vi "laneleftright3.vi"() -> (2 "Coeff right":dbl[](array[numeric]), 3 "Coeff left":dbl[](array[numeric]))   [LabVIEW 2015]
uses:
  <vilib>/Analysis/7linalg.llb/Solve Linear Equations (single right hand).vi
  <vilib>/Analysis/baseanly.llb/Solve Linear Equations By Cholesky.vi
  <vilib>/Analysis/baseanly.llb/Real Matrix to Compact Array.vi
  <vilib>/Analysis/baseanly.llb/Real Compact Tri-Matrix Linear Eqs.vi
  G_LCM.vi
  <vilib>/Analysis/polynomials.llb/1D Polynomial Evaluation (DBL).vi
  G_SEN.vi
  G_ALL.vi
  <vilib>/Analysis/7linalg.llb/Solve Linear Eqs (General).vi
  <vilib>/Analysis/7linalg.llb/Solve Linear Eqs (Gen, single right hand).vi
  <vilib>/Analysis/polynomials.llb/nth Derivative of Polynomial (DBL).vi
  <vilib>/Analysis/polynomials.llb/Polynomial Roots (DBL).vi
  <vilib>/Analysis/polynomials.llb/Scalar Polynomial Evaluation (DBL).vi
  <vilib>/Analysis/1siggen.llb/Ramp Pattern by Delta.vi
  <vilib>/Analysis/NI_AALPro.lvlib
  <vilib>/Analysis/NI_AALBase.lvlib
panel:
  in  "y 2":dbl
  out "fractional index or x 2":dbl
  out "fractional index or x":dbl
  out "range 3":dbl[][](graph)
  out "map_dist":dbl[](array[numeric])
  out "lane_track":dbl[][](array[numeric])
  out "map_track":dbl[][](array[numeric])
  out "lane dist":dbl[](array[numeric])
  out "y_shift":dbl
  out "x_shift":dbl
  out "range 2":dbl[][](graph)
  out "range":dbl[](graph)
  in  "gain":dbl=0.5 min=-1.0 max=1.0
  out "Lane_C_M":dbl[](array[numeric])=[0.8601491478953653, 0.8717844136967624, 0.882947592858927, 0.8936326403234123, 0.9038337699485205, 0.9135454576426009, 0.9227624443554423, 0.9314797389261423, 0.9396926207859084, 0.9473966425143293, 0.9545876322477319, 0.9612616959383189, 0.9674152194628639, 0.9730448705798238, 0.9781476007338057, 0.9827206467064133, 0.9867615321125792, 0.9902680687415704, 0.993238357741943, 0.9956707906498045, 0.9975640502598242, 0.9989171113385246, 0.9997292411794617, 1.0, 0.9997292411794617, 0.9989171113385246, 0.9975640502598242, 0.9956707906498045, 0.993238357741943, 0.9902680687415704, 0.9867615321125792, 0.9827206467064133]
  out "ratio(-1:left1:right)":dbl
  out "NaN/Path/Refnum?":bool
  out "Rleft":dbl
  out "Rright":dbl
  in  "poly":i32=2 min=1 max=4 step=1
  out "Coeff stop":dbl[](array[numeric])
  out "y_end":dbl[](array[numeric])=[0.8601491478953653, 0.8717844136967624, 0.882947592858927, 0.8936326403234123, 0.9038337699485205, 0.9135454576426009, 0.9227624443554423, 0.9314797389261423, 0.9396926207859084, 0.9473966425143293, 0.9545876322477319, 0.9612616959383189, 0.9674152194628639, 0.9730448705798238, 0.9781476007338057, 0.9827206467064133, 0.9867615321125792, 0.9902680687415704, 0.993238357741943, 0.9956707906498045, 0.9975640502598242, 0.9989171113385246, 0.9997292411794617, 1.0, 0.9997292411794617, 0.9989171113385246, 0.9975640502598242, 0.9956707906498045, 0.993238357741943, 0.9902680687415704, 0.9867615321125792, 0.9827206467064133]
  in  "iter":i32=5
  out "Waveform Graph":dbl[](graph)
  out "w":dbl[](array[numeric])
  out "XY Graph 4":cluster{"Y":dbl[], "Y":dbl[]}[](graph)=[{"Y"=array[3210 elements], "Y"=array[3210 elements]}, {"Y"=[-0.0, 0.001154394197769193, 0.004617650635850623, 0.010389990872226917, 0.018471784248973222, 0.02886354801042046, 0.041565947468740205, 0.056579796217107514, 0.0739060563904701, 0.0935458389742223, 0.11550040416098284, 0.13977116175580306, 0.16635967162997645, 0.19526764422393228, 0.2264969410994837, 0.26004957554195585, 0.2959277132125635, 0.3341336728515216, 0.374669927032528, 0.417539102969144, 0.4627439833735707, 0.5102875073687159, 0.560172771454063, 0.6124030305261954, 0.6669816989546717, 0.7239123517142048, 0.7831987255740245, 0.8448447203451934, 0.9088544001870815, 0.975231994973953, 1.0439819017227023, 1.1151086860829622, 1.1886170838907617, 1.2645120027869723, 1.342798523901962, 1.42348190360768, 1.5065675753387922, 1.592061151484188, 1.6799684253507792, 1.770295373200753, 1.8630481563645134, 1.9582331234307588, 2.0558568125157564, 2.1559259536137603, 2.258447471030621], "Y"=[0.0, 0.5, 1.0, 1.5, 2.0, 2.5, 3.0, 3.5, 4.0, 4.5, 5.0, 5.5, 6.0, 6.5, 7.0, 7.5, 8.0, 8.5, 9.0, 9.5, 10.0, 10.5, 11.0, 11.5, 12.0, 12.5, 13.0, 13.5, 14.0, 14.5, 15.0, 15.5, 16.0, 16.5, 17.0, 17.5, 18.0, 18.5, 19.0, 19.5, 20.0, 20.5, 21.0, 21.5, 22.0]}, {"Y"=[0.362252581831572], "Y"=[-0.8199241909738847]}, {"Y"=array[210 elements], "Y"=array[210 elements]}, {"Y"=[-0.925, -0.925, -0.925, -0.6775, -0.6775, -0.925, -0.925, -0.925, -0.925, -0.6775, -0.6775, -0.925, -0.925, -0.925, 0.9025, 0.9025, 0.9025, 0.6775, 0.6775, 0.9025, 0.9025, 0.9025, 0.9025, 0.6775, 0.6775, 0.9025, 0.9025, 0.9025, -0.925], "Y"=[-0.75, -0.224, 0.224, 0.224, -0.224, -0.224, 0.224, 2.415, 2.885, 2.885, 2.415, 2.415, 2.885, 3.5, 3.5, 2.885, 2.415, 2.415, 2.885, 2.885, 2.415, 0.224, -0.224, -0.224, 0.224, 0.224, -0.224, -0.75, -0.75]}, {"Y"=[0.171875, 0.15377271904051304, 0.1346290179491043, 0.11445423440635205, 0.09325870609283447, 0.07105277068912982, 0.04784676587581635, 0.02365102933347224, -0.0015241012573242174, -0.02766828821599482, -0.05477119386196136, -0.08282248051464558, -0.11181181049346922, -0.14172884611785413, -0.17256324970722198, -0.20430468358099463, -0.23694281005859374, -0.27046729145944115, -0.30486779010295867, -0.340133968308568, -0.3762554883956909, -0.41322201268374914, -0.4510232034921646, -0.4896487231403589], "Y"=[0.0, 0.5, 1.0, 1.5, 2.0, 2.5, 3.0, 3.5, 4.0, 4.5, 5.0, 5.5, 6.0, 6.5, 7.0, 7.5, 8.0, 8.5, 9.0, 9.5, 10.0, 10.5, 11.0, 11.5]}, {"Y"=[1.796875, 1.778772719040513, 1.7596290179491043, 1.739454234406352, 1.7182587060928345, 1.6960527706891297, 1.6728467658758164, 1.6486510293334722, 1.6234758987426758, 1.5973317117840051, 1.5702288061380387, 1.5421775194853544, 1.513188189506531, 1.483271153882146, 1.452436750292778, 1.4206953164190055, 1.3880571899414063, 1.354532708540559, 1.3201322098970414, 1.284866031691432, 1.248744511604309, 1.2117779873162509, 1.1739767965078354, 1.135351276859641, 1.0959117660522462, 1.0556686017662287, 1.014632121682167, 0.9728126634806396, 0.9302205648422242, 0.8868661634474992], "Y"=[0.0, 0.5, 1.0, 1.5, 2.0, 2.5, 3.0, 3.5, 4.0, 4.5, 5.0, 5.5, 6.0, 6.5, 7.0, 7.5, 8.0, 8.5, 9.0, 9.5, 10.0, 10.5, 11.0, 11.5, 12.0, 12.5, 13.0, 13.5, 14.0, 14.5]}, {"Y"=[-1.453125, -1.471227280959487, -1.4903709820508957, -1.510545765593648, -1.5317412939071655, -1.5539472293108703, -1.5771532341241836, -1.6013489706665278, -1.6265241012573242, -1.6526682882159949, -1.6797711938619613, -1.7078224805146456, -1.736811810493469, -1.766728846117854, -1.797563249707222, -1.8293046835809945, -1.8619428100585937, -1.895467291459441, -1.9298677901029586], "Y"=[0.0, 0.5, 1.0, 1.5, 2.0, 2.5, 3.0, 3.5, 4.0, 4.5, 5.0, 5.5, 6.0, 6.5, 7.0, 7.5, 8.0, 8.5, 9.0]}, {"Y"=[0.171875, 0.2568230007600336, 0.3384052130063493, 0.44574342526006827, 0.5205081969556753, 0.5917680690742042, 0.659409530134929, 0.7229937549325056, 0.7835496148685115, 0.8405449546633443, 0.9258576868463875], "Y"=[-20.239964538708662, -19.725637940364884, -19.211158961966362, -18.6998967366845, -18.19022720070031, -17.681887266143153, -17.17615515566314, -16.67683575591291, -16.176265245349786, -15.679082775270938, -15.183754484614711]}, {"Y"=[7.134647485270904], "Y"=[38.71960961082238]}, {"Y"=array[980 elements], "Y"=array[980 elements]}, {"Y"=[], "Y"=[]}]
  out "y":dbl[](array[numeric])
  out "x":dbl[](array[numeric])
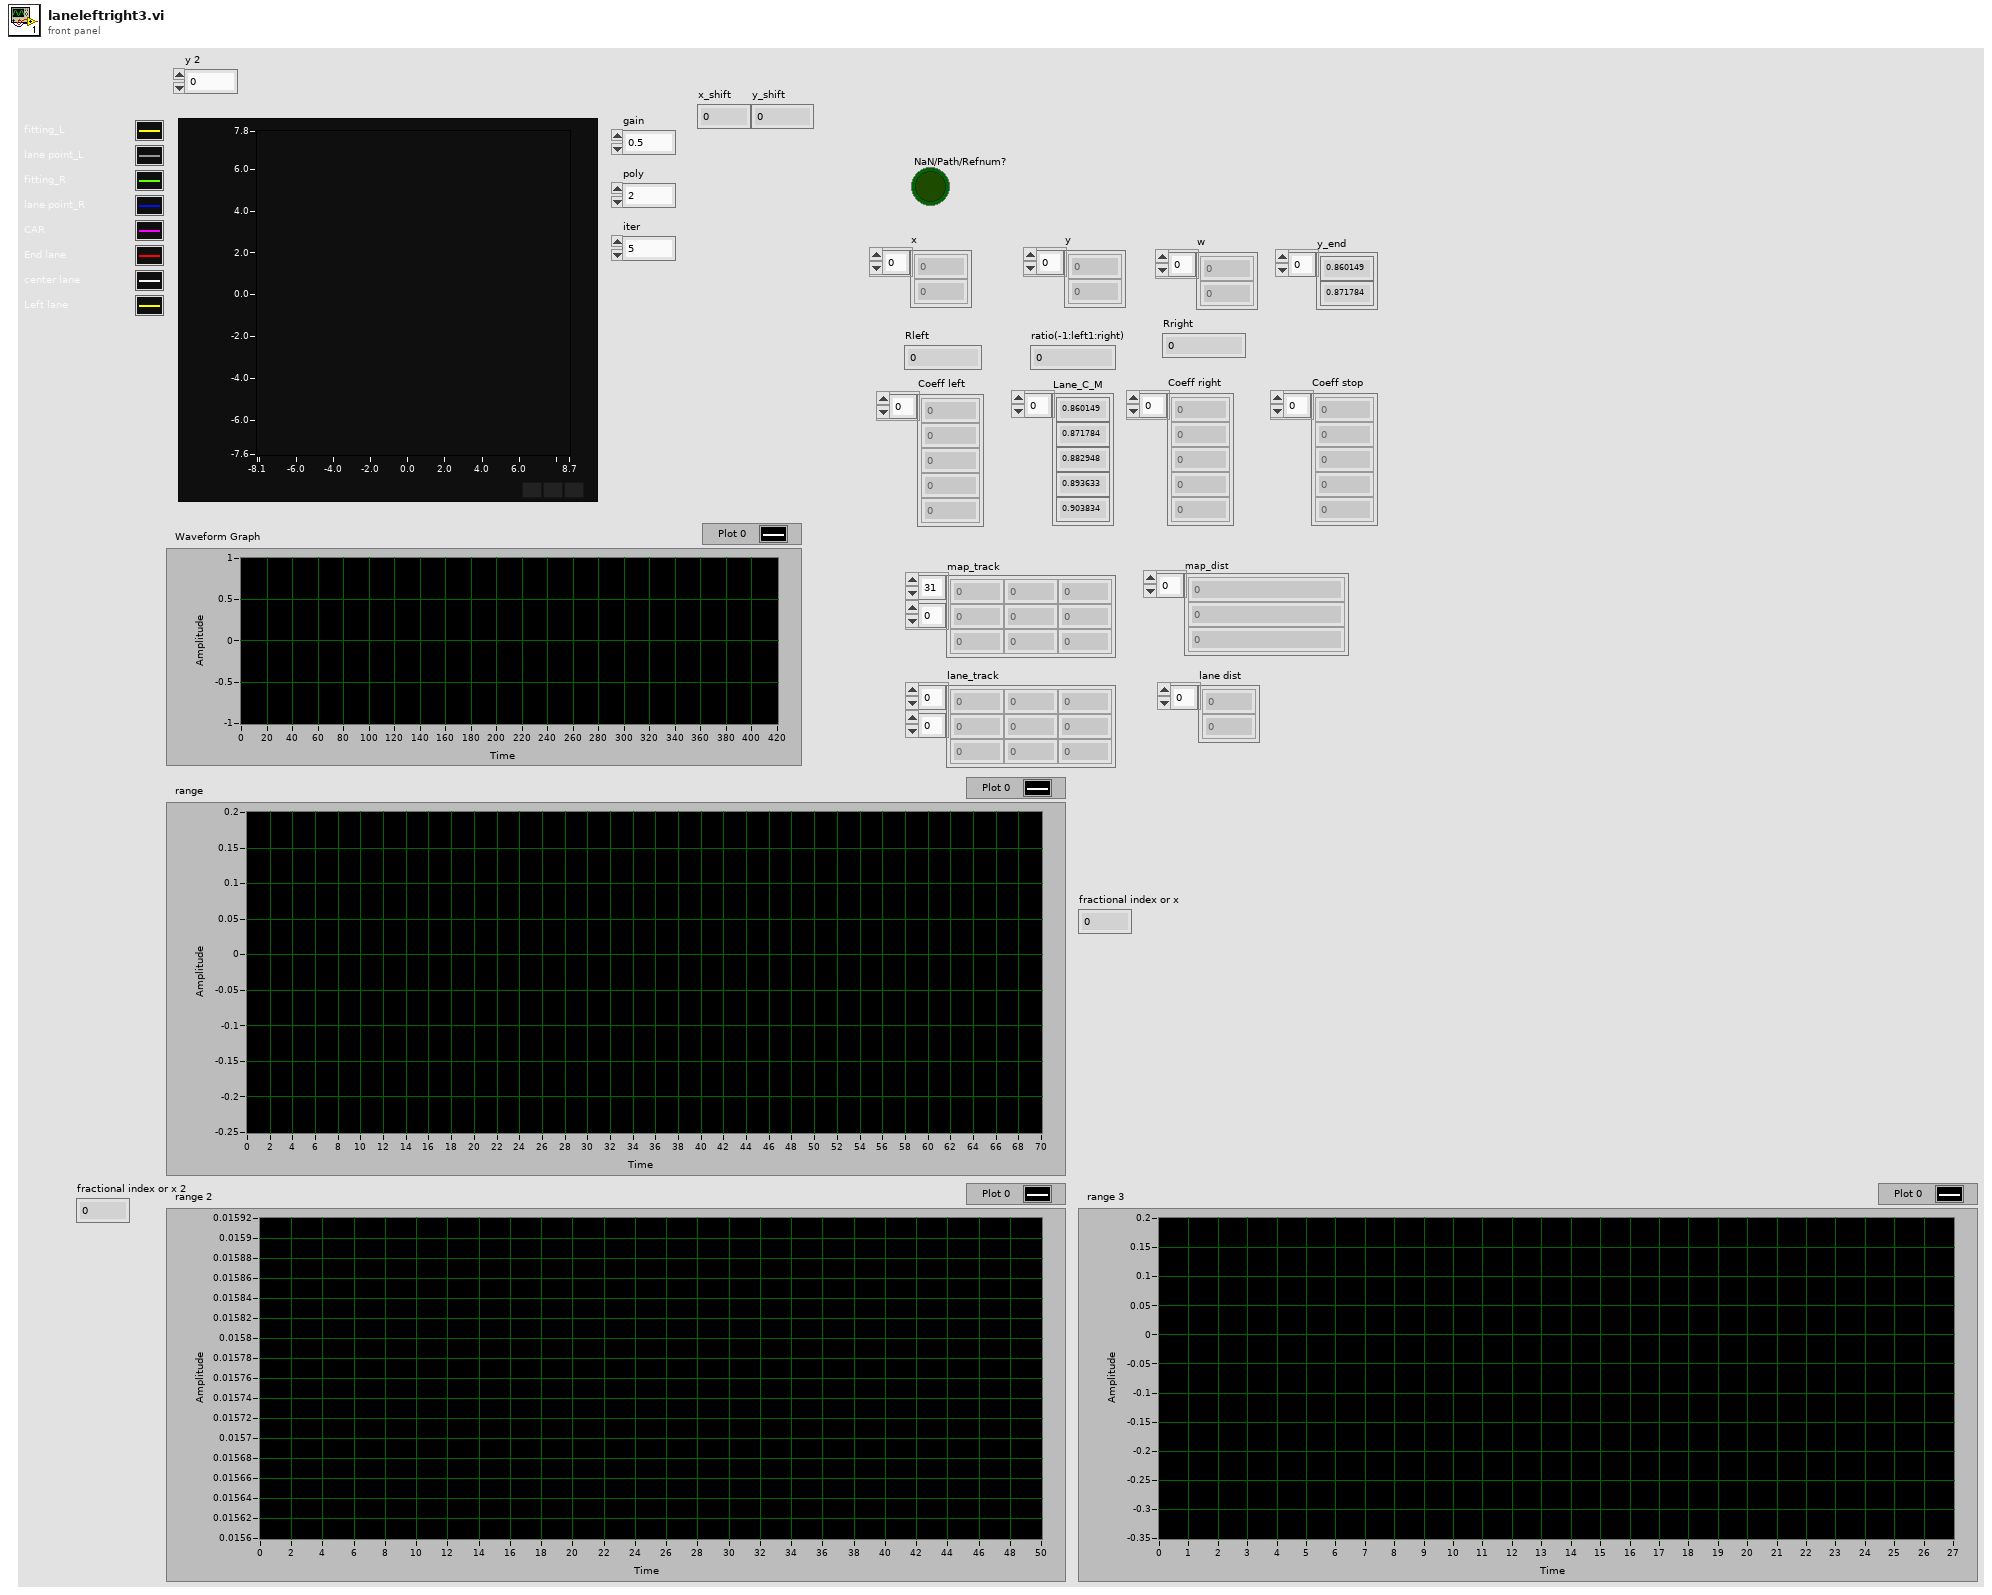
[diagram p1: front panel]
types:
  T1 = cluster{"hash":i64, "sys time":i64, "size":i64, "x":dbl[], "y":dbl[]}
  T2 = cluster{"delta":bool, "Rotational position":dbl, "Rotational position":dbl}[]
  T3 = cluster{"C_Wheel base":dbl, "ratio_steer":dbl, "Overall width":dbl, "af":dbl, "turn radius":dbl, "eval":dbl, "ap":dbl, "an":dbl, "Vmax":dbl, "mu":dbl, "Vlast":dbl}
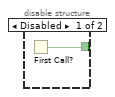
[diagram p2: hidden frame]
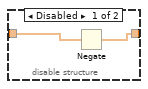
[diagram p3: hidden frame]
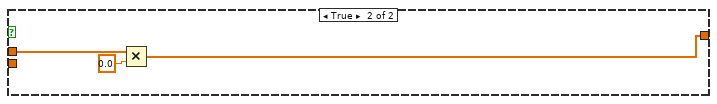
[diagram p4: hidden frame]
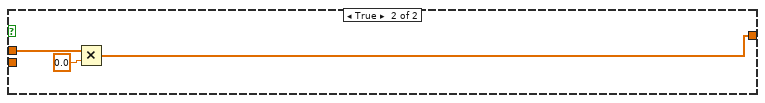
[diagram p5: hidden frame]
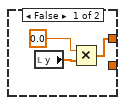
[diagram p6: hidden frame]
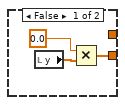
[diagram p7: hidden frame]
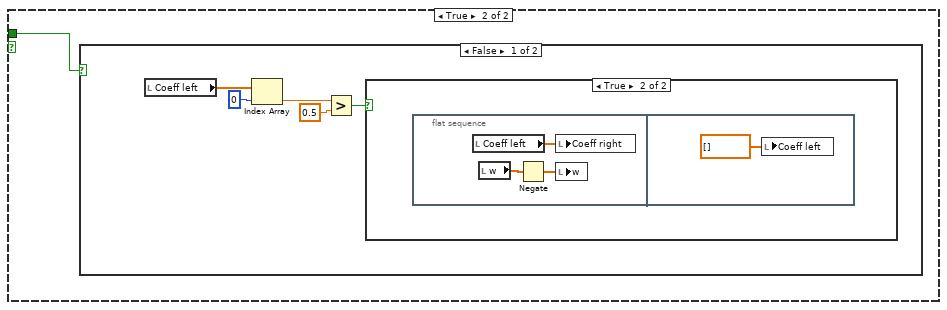
[diagram p12: hidden frame]
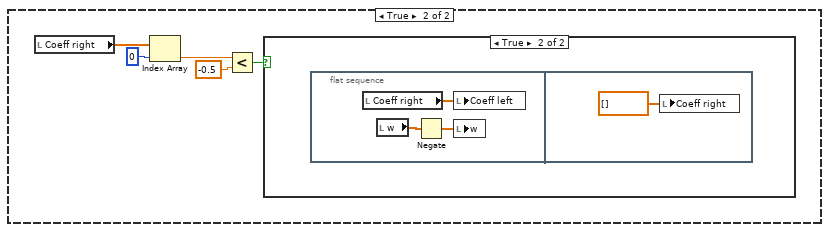
[diagram p14: hidden frame]
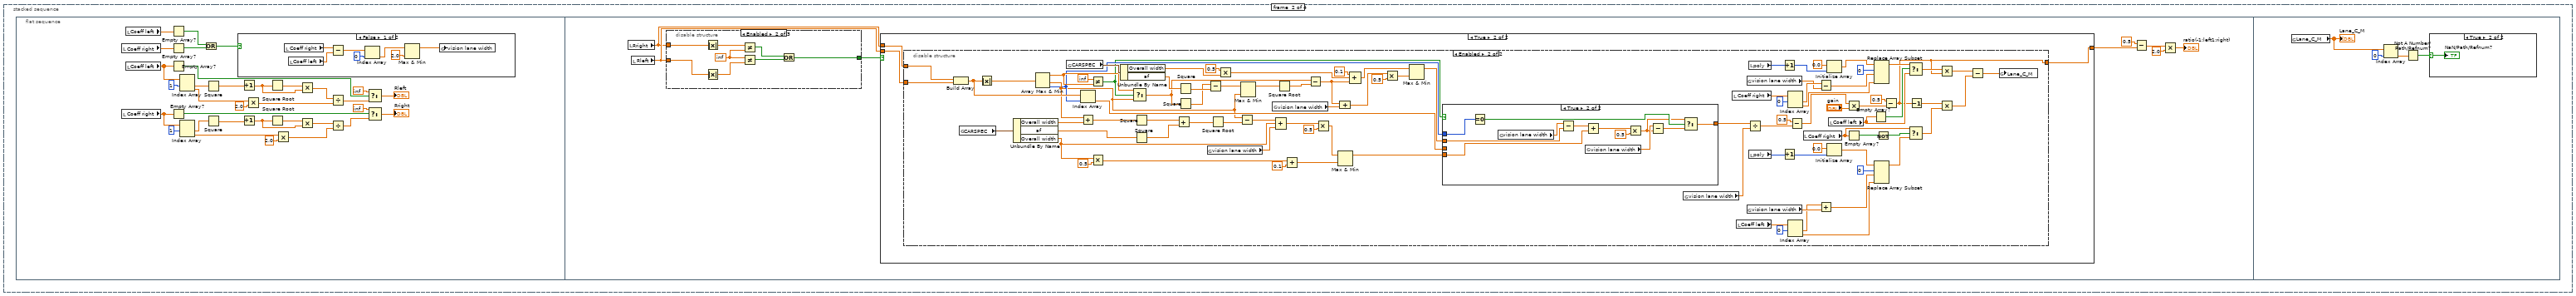
[diagram p16: hidden frame]
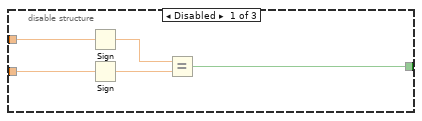
[diagram p18: hidden frame]
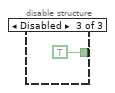
[diagram p19: hidden frame]
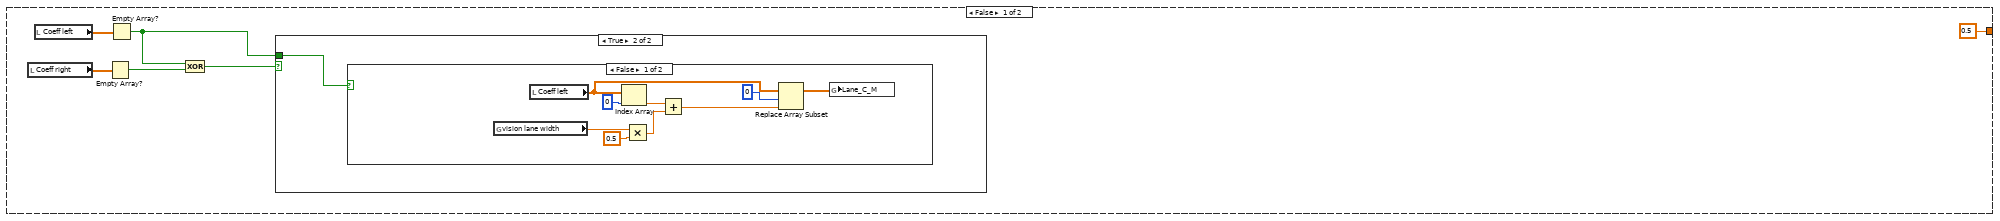
[diagram p20: hidden frame]
diagram:
  n1 = disable-structure shown="Enabled" {
    disable-tunnel: [w2 _] -> w1
    frame Disabled {
      n2 = First Call?() -> (First Call?: T/F=w2:bool)
    }
    frame Enabled {
    }
  }
  n3 = case shown="False" w1 {
    frame False {
      n4 = stacked-sequence {
        frame #0 {
          n5 = flat-sequence {
            frame #0 {
              n6 = global read "G_LCM.vi" "VISION_LANE_PT"() -> (w3:T1)
              n7 = Unbundle By Name(w3) -> ("x"=w20:dbl[], "y"=w14:dbl[])
              n8 = disable-structure shown="Enabled" {
                disable-tunnel: w20 -> [w23 w24]
                disable-tunnel: [w22 w24] -> w21
                frame Disabled {
                  n9 = Negate(x=w23) -> (-x=w22:dbl[])
                }
                frame Enabled {
                }
              }
              n10 = In Range and Coerce(upper limit=10.0 ("delta"), x=w14, lower limit=-10.0) -> (In Range?=w12:bool[])  [unwired: 1 out]
              n11 = Build Cluster Array(w12, w21, w14) -> (w10:T2)
              n12 = Sort 1D Array(array=w10) -> (sorted array=w11:T2)
              n13 = Reverse 1D Array(array=w11) -> (reversed array=w5:T2)
              n14 = for {
                tunnel: w5 -> [w28] mode=indexing
                tunnel: [w27] -> w7 mode=indexing
                tunnel: [w26] -> w8 mode=indexing
                tunnel: [w25] -> w15 mode=indexing
                n15 = Unbundle(w28) -> ("delta"=w25:bool, "Rotational position"=w27:dbl, "Rotational position"=w26:dbl)
              }
              n16 = Boolean To (0,1)(Boolean=w15) -> (0, 1=w6:i16[])
              n17 = Add Array Elements(numeric array=w6) -> (sum=w16:i16)
              n18 = Delete From Array(array=w7, length=w16, index=0) -> (deleted portion=→"x":dbl[])  [unwired: 1 out]
              n19 = Delete From Array(array=w8, length=w16, index=0) -> (deleted portion=→"y":dbl[])  [unwired: 1 out]
            }
            frame #1 {
              n20 = local read "Coeff left"() -> (w60:dbl[])
              n21 = local read "Coeff right"() -> (w59:dbl[])
              n22 = Empty Array?(array=w60) -> (empty?=w61:bool)
              n23 = Empty Array?(array=w59) -> (empty?=w62:bool)
              n24 = local read "y"() -> (w57:dbl[])
              n25 = case shown="False" w61 {
                tunnel: w57 -> [w83 w91]
                tunnel: w60 -> [w80 _]
                tunnel: [w78 w90] -> w58
                frame False {
                  n26 = call-poly <vilib>:"Polynomial Evaluation.vi"("P(x)"=w80, "A"=w83) -> ("P(A)"=w82:dbl[])  [unwired: 1 out]
                  n27 = local read "x"() -> (w81:dbl[])
                  n28 = Subtract(x=w82, y=w81) -> (x-y=w87:dbl[])
                  n29 = Absolute Value(x=w87) -> (abs(x)=w86:dbl[])
                  n30 = Negate(x=w86) -> (-x=w85:dbl[])
                  n31 = Add(x=w85, y=1.0) -> (x+y=w89:dbl[])
                  n32 = Max & Min(x=0.0, y=w89) -> (max(x,y)=w79:dbl[])  [unwired: 1 out]
                  n33 = Negate(x=w79) -> (-x=w78:dbl[])
                }
                frame True {
                  n34 = Multiply(x=w91, y=0.0) -> (x*y=w90:dbl[])
                }
              }
              n35 = local read "x"() -> (w29:dbl[])
              n36 = local read "y"() -> (w63:dbl[])
              n37 = local read "y"() -> (w30:dbl[])
              n38 = case shown="False" w62 {
                tunnel: [w72 w75] -> w55
                tunnel: w59 -> [w71 _]
                tunnel: w63 -> [w64 w76]
                frame False {
                  n39 = call-poly <vilib>:"Polynomial Evaluation.vi"("P(x)"=w71, "A"=w64) -> ("P(A)"=w69:dbl[])  [unwired: 1 out]
                  n40 = local read "x"() -> (w70:dbl[])
                  n41 = Subtract(x=w69, y=w70) -> (x-y=w65:dbl[])
                  n42 = Absolute Value(x=w65) -> (abs(x)=w66:dbl[])
                  n43 = Negate(x=w66) -> (-x=w67:dbl[])
                  n44 = Add(x=w67, y=1.0) -> (x+y=w73:dbl[])
                  n45 = Max & Min(x=0.0, y=w73) -> (max(x,y)=w72:dbl[])  [unwired: 1 out]
                }
                frame True {
                  n46 = Multiply(x=w76, y=0.0) -> (x*y=w75:dbl[])
                }
              }
              n47 = Subtract(x=w29, y=6.0) -> (x-y=w33:dbl[])
              n48 = Subtract(x=w30, y=0.0) -> (x-y=w42:dbl[])
              n49 = Subtract(x=w29, y=-6.0) -> (x-y=w35:dbl[])
              n50 = Square(x=w35) -> (x^2=w34:dbl[])
              n51 = Square(x=w33) -> (x^2=w43:dbl[])
              n52 = Square(x=w42) -> (x^2=w44:dbl[])
              n53 = Add(x=w34, y=w44) -> (x+y=w50:dbl[])
              n54 = Add(x=w44, y=w43) -> (x+y=w45:dbl[])
              n55 = In Range and Coerce(upper limit=36.0, x=w50, lower limit=4.0) -> (In Range?=w52:bool[])  [unwired: 1 out]
              n56 = In Range and Coerce(upper limit=36.0, x=w45, lower limit=4.0) -> (In Range?=w51:bool[])  [unwired: 1 out]
              n57 = Boolean To (0,1)(Boolean=w52) -> (0, 1=w53:i16[])
              n58 = Boolean To (0,1)(Boolean=w51) -> (0, 1=w54:i16[])
              n59 = Multiply(x=i16 -1, y=w53) -> (x*y=w38:i16[])
              n60 = Add(x=w38, y=w54) -> (x+y=w40:i16[])
              n61 = Multiply(x=w40, y=1.0 ("element")) -> (x*y=w56:dbl[])
              n62 = Compound Arithmetic op=ADD(w56, w55, w58) -> (→"w":dbl[])
            }
            frame #2 {
              n63 = for {
                N: "iter" -> [_]
                tunnel: "poly" -> [w96]
                n64 = flat-sequence {
                  tunnel: [w110] -> w102
                  tunnel: w96 -> [w103]
                  tunnel: [w103] -> w95
                  tunnel: [w141] -> w101
                  tunnel: w102 -> [w141]
                  tunnel: [w138] -> w99
                  tunnel: w95 -> [w131]
                  tunnel: w101 -> [w203]
                  tunnel: [w203] -> w100
                  tunnel: w99 -> [w202]
                  tunnel: [w202] -> w98
                  tunnel: [w173] -> w97
                  tunnel: w100 -> [w211]
                  tunnel: w98 -> [w210]
                  tunnel: w97 -> [w209]
                  frame #0 {
                    n65 = local read "w"() -> (w112:dbl[])
                    n66 = Greater?(x=w112, y=0.99) -> (0:w104:bool[])
                    n67 = Boolean To (0,1)(Boolean=w104) -> (0, 1=w105:i16[])
                    n68 = Add Array Elements(numeric array=w105) -> (sum=w108:i16)
                    n69 = Greater?(x=w108, y=i16 50) -> (0:w106:bool)
                    n70 = case shown="True" w106 {
                      tunnel: [w114 w121] -> w110
                      tunnel: [_ w120] -> w109
                      tunnel: w105 -> [_ w117]
                      tunnel: w103 -> [_ w116]
                      frame False {
                        n71 = local read "y"() -> (w115:dbl[])
                        n72 = Multiply(x=0.0, y=w115) -> (x*y=w114:dbl[])
                      }
                      frame True {
                        n73 = local read "x"() -> (w118:dbl[])
                        n74 = local read "y"() -> (w119:dbl[])
                        n75 = call <vilib>:"General Polynomial Fit Coefficients.vi"("Y"=w118, "polynomial order"=w116, "X"=w119, "Weight"=w117) -> ("Polynomial Coefficients"=w120:dbl[])  [unwired: 10 in, 1 out]
                        n76 = local read "y"() -> (w130:dbl[])
                        n77 = call-poly <vilib>:"Polynomial Evaluation.vi"("P(x)"=w120, "A"=w130) -> ("P(A)"=w129:dbl[])  [unwired: 1 out]
                        n78 = local read "x"() -> (w128:dbl[])
                        n79 = Subtract(x=w129, y=w128) -> (x-y=w127:dbl[])
                        n80 = Absolute Value(x=w127) -> (abs(x)=w126:dbl[])
                        n81 = Negate(x=w126) -> (-x=w125:dbl[])
                        n82 = Add(x=w125, y=1.0) -> (x+y=w122:dbl[])
                        n83 = Max & Min(x=0.0, y=w122) -> (max(x,y)=w121:dbl[])  [unwired: 1 out]
                      }
                    }
                    "Coeff right" <- w109
                  }
                  frame #1 {
                    n84 = local read "w"() -> (w139:dbl[])
                    n85 = Less?(x=w139, y=-0.99) -> (x < y?=w134:bool[])
                    n86 = Boolean To (0,1)(Boolean=w134) -> (0, 1=w132:i16[])
                    n87 = Add Array Elements(numeric array=w132) -> (sum=w135:i16)
                    n88 = Greater?(x=w135, y=i16 50) -> (0:w133:bool)
                    n89 = case shown="True" w133 {
                      tunnel: [w142 w150] -> w138
                      tunnel: [_ w149] -> w137
                      tunnel: w132 -> [_ w146]
                      tunnel: w131 -> [_ w145]
                      frame False {
                        n90 = local read "y"() -> (w143:dbl[])
                        n91 = Multiply(x=0.0, y=w143) -> (x*y=w142:dbl[])
                      }
                      frame True {
                        n92 = local read "x"() -> (w147:dbl[])
                        n93 = local read "y"() -> (w148:dbl[])
                        n94 = call <vilib>:"General Polynomial Fit Coefficients.vi"("Y"=w147, "polynomial order"=w145, "X"=w148, "Weight"=w146) -> ("Polynomial Coefficients"=w149:dbl[])  [unwired: 10 in, 1 out]
                        n95 = local read "y"() -> (w154:dbl[])
                        n96 = call-poly <vilib>:"Polynomial Evaluation.vi"("P(x)"=w149, "A"=w154) -> ("P(A)"=w155:dbl[])  [unwired: 1 out]
                        n97 = local read "x"() -> (w156:dbl[])
                        n98 = Subtract(x=w155, y=w156) -> (x-y=w157:dbl[])
                        n99 = Absolute Value(x=w157) -> (abs(x)=w158:dbl[])
                        n100 = Negate(x=w158) -> (-x=w152:dbl[])
                        n101 = Add(x=w152, y=1.0) -> (x+y=w159:dbl[])
                        n102 = Max & Min(x=0.0, y=w159) -> (max(x,y)=w153:dbl[])  [unwired: 1 out]
                        n103 = Negate(x=w153) -> (-x=w150:dbl[])
                      }
                    }
                    "Coeff left" <- w137
                  }
                  frame #2 {
                    n104 = local read "w"() -> (w181:dbl[])
                    n105 = Absolute Value(x=w181) -> (abs(x)=w180:dbl[])
                    n106 = local read "y"() -> (w185:dbl[])
                    n107 = Greater?(x=w185, y=2.0) -> (0:w183:bool[])
                    n108 = Less?(x=w180, y=0.25) -> (x < y?=w179:bool[])
                    n109 = And(x=w183, y=w179) -> (x .and. y?=w182:bool[])
                    n110 = Boolean To (0,1)(Boolean=w182) -> (0, 1=w201:i16[])
                    n111 = local read "y"() -> (w195:dbl[])
                    n112 = local read "x"() -> (w194:dbl[])
                    n113 = call <vilib>:"General Polynomial Fit Coefficients.vi"("Y"=w195, "polynomial order"=1, "X"=w194, "Weight"=w201) -> ("Polynomial Coefficients"=w166:dbl[])  [unwired: 10 in, 1 out]
                    n114 = local read "x"() -> (w199:dbl[])
                    n115 = Equal To 0?(x=w166) -> (x = 0?=w165:bool[])
                    n116 = Index Array(array=w166, index=1) -> (element=w176:dbl)
                    n117 = call-poly <vilib>:"Polynomial Evaluation.vi"("P(x)"=w166, "A"=w199) -> ("P(A)"=w198:dbl[])  [unwired: 1 out]
                    n118 = And Array Elements(Boolean array=w165) -> (logical AND=w162:bool)
                    n119 = In Range and Coerce(upper limit=0.5, x=w176, lower limit=-0.5) -> (In Range?=w164:bool)  [unwired: 1 out]
                    n120 = Not(x=w162) -> (.not. x?=w161:bool)
                    n121 = local read "y"() -> (w197:dbl[])
                    n122 = Subtract(x=w198, y=w197) -> (x-y=w196:dbl[])
                    n123 = disable-structure shown="Enabled" {
                      disable-tunnel: w164 -> [w206 _]
                      disable-tunnel: [w205 _] -> w163
                      disable-tunnel: w161 -> [w204 _]
                      frame Enabled {
                        n124 = And(x=w204, y=w206) -> (x .and. y?=w205:bool)
                      }
                      frame Disabled {
                      }
                    }
                    n125 = Absolute Value(x=w196) -> (abs(x)=w193:dbl[])
                    n126 = Greater?(x=w193, y=0.25 ("Numeric 2")) -> (0:w191:bool[])
                    n127 = Not(x=w191) -> (.not. x?=w190:bool[])
                    n128 = Boolean To (0,1)(Boolean=w191) -> (0, 1=w186:i16[])
                    n129 = Boolean To (0,1)(Boolean=w190) -> (0, 1=w189:i16[])
                    n130 = Select(t=w166, s=w163, f=dbl[] []) -> (s? t:f=→"Coeff stop":dbl[])
                    n131 = Multiply(x=w189, y=0.5) -> (x*y=w187:dbl[])
                    n132 = Add(x=w186, y=w187) -> (x+y=w172:dbl[])
                    n133 = Multiply(x=w172, y=0.0) -> (x*y=w170:dbl[])
                    n134 = Increment(x=w170) -> (x+1=w169:dbl[])
                    n135 = Select(t=w172, s=w163, f=w169) -> (s? t:f=w173:dbl[])
                  }
                  frame #3 {
                    n136 = local read "w"() -> (w215:dbl[])
                    n137 = Compound Arithmetic op=ADD(w215, w211, w210) -> (w208:dbl[])
                    n138 = Multiply(x=w209, y=w208) -> (x*y=w207:dbl[])
                    n139 = In Range and Coerce(upper limit=1.0, x=w207, lower limit=-1.0) -> (coerced(x)=w212:dbl[])  [unwired: 1 out]
                    n140 = local write "w"(w212) -> ()
                  }
                }
              }
            }
            frame #3 {
              n141 = disable-structure shown="Enabled" {
                disable-tunnel: [w219 _] -> w216
                frame Enabled {
                  n142 = local read "Coeff left"() -> (w218:dbl[])
                  n143 = Index Array(array=w218, index=1) -> (element=w221:dbl)
                  n144 = Absolute Value(x=w221) -> (abs(x)=w222:dbl)
                  n145 = Less?(x=w222, y=1.0) -> (x < y?=w224:bool)
                  n146 = Select(t=w218, s=w224, f=dbl[] []) -> (s? t:f=w219:dbl[])
                }
                frame Disabled {
                }
              }
              n147 = disable-structure shown="Enabled" {
                disable-tunnel: [w228 _] -> w217
                frame Enabled {
                  n148 = local read "Coeff right"() -> (w226:dbl[])
                  n149 = Index Array(array=w226, index=1) -> (element=w232:dbl)
                  n150 = Absolute Value(x=w232) -> (abs(x)=w231:dbl)
                  n151 = Less?(x=w231, y=1.0) -> (x < y?=w229:bool)
                  n152 = Select(t=w226, s=w229, f=dbl[] []) -> (s? t:f=w228:dbl[])
                }
                frame Disabled {
                }
              }
              n153 = local write "Coeff left"(w216) -> ()
              n154 = local write "Coeff right"(w217) -> ()
            }
            frame #4 {
              n155 = local read "Coeff right"() -> (w235:dbl[])
              n156 = local read "Coeff left"() -> (w234:dbl[])
              n157 = Empty Array?(array=w235) -> (empty?=w236:bool)
              n158 = Empty Array?(array=w234) -> (empty?=w238:bool)
              n159 = Exclusive Or(1:w236, 2:w238) -> (0:w237:bool)
              n160 = case shown="False" w237 {
                tunnel: w238 -> [_ w258]
                frame False {
                  n161 = local read "Coeff right"() -> (w242:dbl[])
                  n162 = local read "Coeff left"() -> (w243:dbl[])
                  n163 = Index Array(array=w243) -> (element=w241:dbl)  [unwired: 1 in]
                  n164 = Index Array(array=w242) -> (element=w240:dbl)  [unwired: 1 in]
                  n165 = Greater?(x=w241, y=w240) -> (0:w239:bool)
                  n166 = case shown="True" w239 {
                    frame False {
                    }
                    frame True {
                      n167 = flat-sequence {
                        tunnel: [w251] -> w247
                        tunnel: [w250] -> w246
                        tunnel: [w249] -> w245
                        tunnel: [w255] -> w248
                        tunnel: w247 -> [w255]
                        tunnel: w246 -> [w254]
                        tunnel: w245 -> [w253]
                        tunnel: [w252] -> w244
                        tunnel: w248 -> [w257]
                        tunnel: w244 -> [w256]
                        frame #0 {
                          n168 = local read "Coeff right"() -> (w251:dbl[])
                          n169 = local read "Coeff left"() -> (w250:dbl[])
                          n170 = local read "w"() -> (w249:dbl[])
                        }
                        frame #1 {
                          n171 = local write "Coeff right"(w254) -> ()
                          n172 = Negate(x=w253) -> (-x=w252:dbl[])
                        }
                        frame #2 {
                          n173 = local write "w"(w256) -> ()
                          n174 = local write "Coeff left"(w257) -> ()
                        }
                      }
                    }
                  }
                }
                frame True {
                  n175 = case shown="False" w258 {
                    frame False {
                      n176 = local read "Coeff left"() -> (w263:dbl[])
                      n177 = Index Array(array=w263, index=0) -> (element=w261:dbl)
                      n178 = Greater?(x=w261, y=0.5) -> (0:w259:bool)
                      n179 = case shown="True" w259 {
                        frame False {
                        }
                        frame True {
                          n180 = flat-sequence {
                            frame #0 {
                              n181 = local read "Coeff left"() -> (w266:dbl[])
                              n182 = local read "w"() -> (w265:dbl[])
                              n183 = Negate(x=w265) -> (-x=w264:dbl[])
                              n184 = local write "Coeff right"(w266) -> ()
                              n185 = local write "w"(w264) -> ()
                            }
                            frame #1 {
                              n186 = local write "Coeff left"(dbl[] []) -> ()
                            }
                          }
                        }
                      }
                    }
                    frame True {
                      n187 = local read "Coeff right"() -> (w272:dbl[])
                      n188 = Index Array(array=w272, index=0) -> (element=w270:dbl)
                      n189 = Less?(x=w270, y=-0.5) -> (x < y?=w268:bool)
                      n190 = case shown="True" w268 {
                        frame False {
                        }
                        frame True {
                          n191 = flat-sequence {
                            frame #0 {
                              n192 = local read "Coeff right"() -> (w275:dbl[])
                              n193 = local read "w"() -> (w274:dbl[])
                              n194 = Negate(x=w274) -> (-x=w273:dbl[])
                              n195 = local write "Coeff left"(w275) -> ()
                              n196 = local write "w"(w273) -> ()
                            }
                            frame #1 {
                              n197 = local write "Coeff right"(dbl[] []) -> ()
                            }
                          }
                        }
                      }
                    }
                  }
                }
              }
            }
            frame #5 {
              n198 = local read "Coeff right"() -> (w278:dbl[])
              n199 = local read "Coeff left"() -> (w277:dbl[])
              n200 = global write "G_SEN.vi" "Lane_L_M"(w277) -> ()
              n201 = global write "G_SEN.vi" "Lane_R_M"(w278) -> ()
            }
          }
        }
        frame #1 {
          n202 = flat-sequence {
            frame #0 {
              n203 = local read "Coeff right"() -> (w280:dbl[])
              n204 = local read "Coeff right"() -> (w308:dbl[])
              n205 = local read "Coeff left"() -> (w279:dbl[])
              n206 = local read "Coeff left"() -> (w306:dbl[])
              n207 = Empty Array?(array=w279) -> (empty?=w282:bool)
              n208 = Empty Array?(array=w280) -> (empty?=w283:bool)
              n209 = Empty Array?(array=w306) -> (empty?=w300:bool)
              n210 = Empty Array?(array=w308) -> (empty?=w302:bool)
              n211 = Index Array(array=w306, index #1=1 ("index")) -> (element #1=w299:dbl, element #2=w292:dbl)  [unwired: 1 in]
              n212 = Index Array(array=w308, index #1=1 ("index")) -> (element #1=w284:dbl, element #2=w291:dbl)  [unwired: 1 in]
              n213 = Or(x=w282, y=w283) -> (x .or. y?=w281:bool)
              n214 = Square(x=w299) -> (x^2=w298:dbl)
              n215 = Square(x=w284) -> (x^2=w285:dbl)
              n216 = case shown="False" w281 {
                frame False {
                  n217 = local read "Coeff right"() -> (w315:dbl[])
                  n218 = local read "Coeff left"() -> (w312:dbl[])
                  n219 = Subtract(x=w315, y=w312) -> (x-y=w313:dbl[])
                  n220 = Index Array(array=w313, index=0) -> (element=w316:dbl)
                  n221 = Max & Min(x=w316, y=2.0) -> (max(x,y)=w317:dbl)  [unwired: 1 out]
                  n222 = global write "G_SEN.vi" "vision lane width"(w317) -> ()
                }
                frame True {
                }
              }
              n223 = Increment(x=w298) -> (x+1=w296:dbl)
              n224 = Increment(x=w285) -> (x+1=w287:dbl)
              n225 = Multiply(x=w292, y=2.0) -> (x*y=w294:dbl)
              n226 = Square Root(x=w296) -> (sqrt(x)=w297:dbl)
              n227 = Square Root(x=w287) -> (sqrt(x)=w286:dbl)
              n228 = Multiply(x=w291, y=2.0) -> (x*y=w289:dbl)
              n229 = Multiply(x=w297, y=w296) -> (x*y=w295:dbl)
              n230 = Multiply(x=w286, y=w287) -> (x*y=w288:dbl)
              n231 = Divide(x=w295, y=w294) -> (x/y=w301:dbl)
              n232 = Divide(x=w288, y=w289) -> (x/y=w303:dbl)
              n233 = Select(t=inf, s=w300, f=w301) -> (s? t:f=→"Rleft":dbl)
              n234 = Select(t=inf, s=w302, f=w303) -> (s? t:f=→"Rright":dbl)
            }
            frame #1 {
              n235 = local read "Rright"() -> (w319:dbl)
              n236 = local read "Rleft"() -> (w320:dbl)
              n237 = disable-structure shown="Enabled" {
                disable-tunnel: w319 -> [w331 w338 _]
                disable-tunnel: w320 -> [w330 w339 _]
                disable-tunnel: [w327 w334 TRUE] -> w321
                frame Disabled {
                  n238 = Sign(1:w331) -> (0:w329:dbl)
                  n239 = Sign(1:w330) -> (0:w328:dbl)
                  n240 = Equal?(x=w329, y=w328) -> (x = y?=w327:bool)
                }
                frame Enabled {
                  w336 = inf
                  n241 = Absolute Value(x=w338) -> (abs(x)=w337:dbl)
                  n242 = Absolute Value(x=w339) -> (abs(x)=w335:dbl)
                  n243 = Not Equal?(x=w337, y=w336) -> (x != y?=w333:bool)
                  n244 = Not Equal?(x=w336, y=w335) -> (x != y?=w332:bool)
                  n245 = Or(x=w333, y=w332) -> (x .or. y?=w334:bool)
                }
                frame Disabled {
                }
              }
              n246 = case shown="True" w321 {
                tunnel: w319 -> [_ w376]
                tunnel: w320 -> [_ w375]
                tunnel: [0.5 w374] -> w322
                frame False {
                  n247 = local read "Coeff right"() -> (w345:dbl[])
                  n248 = local read "Coeff left"() -> (w346:dbl[])
                  n249 = Empty Array?(array=w345) -> (empty?=w344:bool)
                  n250 = Empty Array?(array=w346) -> (empty?=w342:bool)
                  n251 = Exclusive Or(1:w344, 2:w342) -> (0:w343:bool)
                  n252 = case shown="True" w343 {
                    tunnel: w342 -> [w347 w355]
                    frame False {
                      n253 = case shown="True" w347 {
                        frame False {
                          w348 = 0.5
                          n254 = local read "Coeff right"() -> (w352:dbl[])
                          n255 = local read "Coeff left"() -> (w354:dbl[])
                          n256 = Decrement(x=w348) -> (x-1=w353:dbl)
                          n257 = Multiply(x=w354, y=w348) -> (x*y=w351:dbl[])
                          n258 = Multiply(x=w353, y=w352) -> (x*y=w350:dbl[])
                          n259 = Subtract(x=w351, y=w350) -> (x-y=w349:dbl[])
                          n260 = global write "G_SEN.vi" "Lane_C_M"(w349) -> ()
                        }
                        frame True {
                        }
                      }
                    }
                    frame True {
                      n261 = case shown="False" w355 {
                        frame False {
                          n262 = global read "G_SEN.vi" "vision lane width"() -> (w358:dbl)
                          n263 = local read "Coeff left"() -> (w364:dbl[])
                          n264 = Index Array(array=w364, index=0) -> (element=w362:dbl)
                          n265 = Multiply(x=w358, y=0.5) -> (x*y=w356:dbl)
                          n266 = Add(x=w362, y=w356) -> (x+y=w361:dbl)
                          n267 = Replace Array Subset(array=w364, new element=w361, index=0) -> (w359:dbl[])
                          n268 = global write "G_SEN.vi" "Lane_C_M"(w359) -> ()
                        }
                        frame True {
                          n269 = global read "G_SEN.vi" "vision lane width"() -> (w367:dbl)
                          n270 = local read "Coeff right"() -> (w373:dbl[])
                          n271 = Index Array(array=w373, index=0) -> (element=w371:dbl)
                          n272 = Multiply(x=w367, y=0.5) -> (x*y=w365:dbl)
                          n273 = Subtract(x=w371, y=w365) -> (x-y=w370:dbl)
                          n274 = Replace Array Subset(array=w373, new element=w370, index=0) -> (w368:dbl[])
                          n275 = global write "G_SEN.vi" "Lane_C_M"(w368) -> ()
                        }
                      }
                    }
                  }
                }
                frame True {
                  n276 = disable-structure shown="Enabled" {
                    disable-tunnel: w376 -> [w385 w609]
                    disable-tunnel: w375 -> [w384 w608]
                    disable-tunnel: [_ w536] -> w374
                    frame Disabled {
                      n277 = Absolute Value(x=w385) -> (abs(x)=w407:dbl)
                      n278 = Absolute Value(x=w384) -> (abs(x)=w406:dbl)
                      n279 = global read "G_ALL.vi" "CARSPEC"() -> (w402:T3)
                      n280 = global read "G_ALL.vi" "CARSPEC"() -> (w423:T3)
                      n281 = Build Array(w407, w406) -> (w405:dbl[])
                      n282 = Unbundle By Name(w402) -> ("af"=w401:dbl, "Overall width"=w391:dbl)
                      n283 = Unbundle By Name(w423) -> ("Overall width"=w412:dbl, "af"=w420:dbl, "Overall width"=w408:dbl)
                      n284 = Array Max & Min(array=w405) -> (min value=w398:dbl, min index (indices)=w404:i32)  [unwired: 2 out]
                      n285 = Add(x=w398, y=w412) -> (x+y=w422:dbl)
                      n286 = Square(x=w398) -> (x^2=w389:dbl)
                      n287 = Square(x=w401) -> (x^2=w388:dbl)
                      n288 = Multiply(x=w391, y=0.5) -> (x*y=w390:dbl)
                      n289 = Square(x=w422) -> (x^2=w421:dbl)
                      n290 = Square(x=w420) -> (x^2=w413:dbl)
                      n291 = Subtract(x=w389, y=w388) -> (x-y=w383:dbl)
                      n292 = Multiply(x=w408, y=0.5) -> (x*y=w409:dbl)
                      n293 = Add(x=w421, y=w413) -> (x+y=w419:dbl)
                      n294 = Square Root(x=w383) -> (sqrt(x)=w400:dbl)
                      n295 = global read "G_SEN.vi" "vision lane width"() -> (w394:dbl)
                      n296 = global read "G_SEN.vi" "vision lane width"() -> (w418:dbl)
                      n297 = Subtract(x=w400, y=w391) -> (x-y=w399:dbl)
                      n298 = Square Root(x=w419) -> (sqrt(x)=w417:dbl)
                      n299 = Subtract(x=w398, y=w399) -> (x-y=w393:dbl)
                      n300 = Subtract(x=w417, y=w398) -> (x-y=w416:dbl)
                      n301 = Subtract(x=w394, y=w393) -> (x-y=w395:dbl)
                      n302 = Subtract(x=w418, y=w416) -> (x-y=w415:dbl)
                      n303 = global read "G_SEN.vi" "vision lane width"() -> (w379:dbl)
                      n304 = global read "G_SEN.vi" "vision lane width"() -> (w386:dbl)
                      n305 = Multiply(x=w395, y=0.5) -> (x*y=w397:dbl)
                      n306 = Multiply(x=w415, y=0.5) -> (x*y=w410:dbl)
                      n307 = Compound Arithmetic op=ADD(w397, w390) -> (w387:dbl)
                      n308 = Compound Arithmetic op=ADD(w410, w409) -> (w403:dbl)
                      n309 = Subtract(x=w386, y=w387) -> (x-y=w381:dbl)
                      n310 = Less Than 0?(x=w383) -> (x < 0?=w382:bool)
                      n311 = Multiply(x=0.5 ("y"), y=w379) -> (x*y=w378:dbl)
                      n312 = Select(t=w378, s=w382, f=w381) -> (s? t:f=w380:dbl)
                      n313 = case shown="1" w404 {
                        tunnel: w403 -> [w425 w473]
                        tunnel: w380 -> [w424 w471]
                        frame 0, Default {
                          n314 = local read "Rright"() -> (w427:dbl)
                          n315 = Greater Than 0?(x=w427) -> (x > 0?=w426:bool)
                          n316 = case shown="True" w426 {
                            tunnel: w425 -> [_ w448]
                            tunnel: w424 -> [w430 w447]
                            frame False {
                              n317 = local read "Coeff left"() -> (w429:dbl[])
                              n318 = Empty Array?(array=w429) -> (empty?=w428:bool)
                              n319 = case shown="False" w428 {
                                tunnel: w430 -> [w431 w440]
                                frame False {
                                n320 = global read "G_SEN.vi" "vision lane width"() -> (w439:dbl)
                                n321 = Divide(x=w431, y=w439) -> (x/y=w437:dbl)
                                n322 = local read "Coeff right"() -> (w435:dbl[])
                                n323 = local read "Coeff left"() -> (w438:dbl[])
                                n324 = Decrement(x=w437) -> (x-1=w436:dbl)
                                n325 = Multiply(x=w438, y=w437) -> (x*y=w434:dbl[])
                                n326 = Multiply(x=w436, y=w435) -> (x*y=w433:dbl[])
                                n327 = Subtract(x=w434, y=w433) -> (x-y=w432:dbl[])
                                n328 = global write "G_SEN.vi" "Lane_C_M"(w432) -> ()
                                }
                                frame True {
                                n329 = local read "Coeff right"() -> (w446:dbl[])
                                n330 = Index Array(array=w446, index=0) -> (element=w444:dbl)
                                n331 = Subtract(x=w444, y=w440) -> (x-y=w443:dbl)
                                n332 = Replace Array Subset(array=w446, new element=w443, index=0) -> (w441:dbl[])
                                n333 = global write "G_SEN.vi" "Lane_C_M"(w441) -> ()
                                }
                              }
                            }
                            frame True {
                              n334 = local read "Coeff left"() -> (w450:dbl[])
                              n335 = Empty Array?(array=w450) -> (empty?=w449:bool)
                              n336 = case shown="False" w449 {
                                tunnel: w448 -> [w454 w464]
                                tunnel: w447 -> [w455 _]
                                frame False {
                                n337 = Add(x=w455, y=w454) -> (x+y=w453:dbl)
                                n338 = global read "G_SEN.vi" "vision lane width"() -> (w463:dbl)
                                n339 = Multiply(x=w453, y=0.5) -> (x*y=w451:dbl)
                                n340 = Divide(x=w451, y=w463) -> (x/y=w461:dbl)
                                n341 = local read "Coeff right"() -> (w459:dbl[])
                                n342 = local read "Coeff left"() -> (w462:dbl[])
                                n343 = Decrement(x=w461) -> (x-1=w460:dbl)
                                n344 = Multiply(x=w462, y=w461) -> (x*y=w458:dbl[])
                                n345 = Multiply(x=w460, y=w459) -> (x*y=w457:dbl[])
                                n346 = Subtract(x=w458, y=w457) -> (x-y=w456:dbl[])
                                n347 = global write "G_SEN.vi" "Lane_C_M"(w456) -> ()
                                }
                                frame True {
                                n348 = local read "Coeff right"() -> (w470:dbl[])
                                n349 = Index Array(array=w470, index=0) -> (element=w468:dbl)
                                n350 = Subtract(x=w468, y=w464) -> (x-y=w467:dbl)
                                n351 = Replace Array Subset(array=w470, new element=w467, index=0) -> (w465:dbl[])
                                n352 = global write "G_SEN.vi" "Lane_C_M"(w465) -> ()
                                }
                              }
                            }
                          }
                        }
                        frame 1 {
                          n353 = local read "Rleft"() -> (w474:dbl)
                          n354 = Less Than 0?(x=w474) -> (x < 0?=w472:bool)
                          n355 = case shown="True" w472 {
                            tunnel: w473 -> [_ w495]
                            tunnel: w471 -> [w477 w494]
                            frame False {
                              n356 = local read "Coeff right"() -> (w476:dbl[])
                              n357 = Empty Array?(array=w476) -> (empty?=w475:bool)
                              n358 = case shown="False" w475 {
                                tunnel: w477 -> [w478 w487]
                                frame False {
                                n359 = global read "G_SEN.vi" "vision lane width"() -> (w486:dbl)
                                n360 = Divide(x=w478, y=w486) -> (x/y=w484:dbl)
                                n361 = local read "Coeff right"() -> (w485:dbl[])
                                n362 = local read "Coeff left"() -> (w482:dbl[])
                                n363 = Decrement(x=w484) -> (x-1=w483:dbl)
                                n364 = Multiply(x=w485, y=w484) -> (x*y=w481:dbl[])
                                n365 = Multiply(x=w483, y=w482) -> (x*y=w480:dbl[])
                                n366 = Subtract(x=w481, y=w480) -> (x-y=w479:dbl[])
                                n367 = global write "G_SEN.vi" "Lane_C_M"(w479) -> ()
                                }
                                frame True {
                                n368 = local read "Coeff left"() -> (w493:dbl[])
                                n369 = Index Array(array=w493, index=0) -> (element=w491:dbl)
                                n370 = Add(x=w491, y=w487) -> (x+y=w490:dbl)
                                n371 = Replace Array Subset(array=w493, new element=w490, index=0) -> (w488:dbl[])
                                n372 = global write "G_SEN.vi" "Lane_C_M"(w488) -> ()
                                }
                              }
                            }
                            frame True {
                              n373 = local read "Coeff right"() -> (w497:dbl[])
                              n374 = Empty Array?(array=w497) -> (empty?=w496:bool)
                              n375 = case shown="False" w496 {
                                tunnel: w495 -> [w499 w511]
                                tunnel: w494 -> [w500 _]
                                frame False {
                                n376 = Add(x=w500, y=w499) -> (x+y=w502:dbl)
                                n377 = global read "G_SEN.vi" "vision lane width"() -> (w510:dbl)
                                n378 = Multiply(x=w502, y=0.5) -> (x*y=w498:dbl)
                                n379 = Divide(x=w498, y=w510) -> (x/y=w508:dbl)
                                n380 = local read "Coeff right"() -> (w509:dbl[])
                                n381 = local read "Coeff left"() -> (w506:dbl[])
                                n382 = Decrement(x=w508) -> (x-1=w507:dbl)
                                n383 = Multiply(x=w509, y=w508) -> (x*y=w505:dbl[])
                                n384 = Multiply(x=w507, y=w506) -> (x*y=w504:dbl[])
                                n385 = Subtract(x=w505, y=w504) -> (x-y=w503:dbl[])
                                n386 = global write "G_SEN.vi" "Lane_C_M"(w503) -> ()
                                }
                                frame True {
                                n387 = local read "Coeff left"() -> (w517:dbl[])
                                n388 = Index Array(array=w517, index=0) -> (element=w515:dbl)
                                n389 = Add(x=w515, y=w511) -> (x+y=w514:dbl)
                                n390 = Replace Array Subset(array=w517, new element=w514, index=0) -> (w512:dbl[])
                                n391 = global write "G_SEN.vi" "Lane_C_M"(w512) -> ()
                                }
                              }
                            }
                          }
                        }
                      }
                    }
                    frame Enabled {
                      n392 = Build Array(w609, w608) -> (w583:dbl[])
                      n393 = global read "G_ALL.vi" "CARSPEC"() -> (w606:T3)
                      n394 = Absolute Value(x=w583) -> (abs(x)=w607:dbl[])
                      n395 = Unbundle By Name(w606) -> ("Overall width"=w605:dbl, "af"=w603:dbl, "Overall width"=w531:dbl)
                      n396 = Array Max & Min(array=w607) -> (max value=w585:dbl, min value=w541:dbl, min index (indices)=w582:i32)  [unwired: 1 out]
                      n397 = global read "G_ALL.vi" "CARSPEC"() -> (w594:T3)
                      n398 = Index Array(array=w583, index=w582) -> (element=w581:dbl)
                      n399 = Add(x=w541, y=w605) -> (x+y=w604:dbl)
                      n400 = Not Equal?(x=inf, y=w585) -> (x != y?=w580:bool)
                      n401 = Multiply(x=w531, y=0.5) -> (x*y=w530:dbl)
                      n402 = Unbundle By Name(w594) -> ("Overall width"=w525:dbl, "af"=w593:dbl)
                      n403 = Select(t=w585, s=w580, f=w541) -> (s? t:f=w584:dbl)
                      n404 = Square(x=w604) -> (x^2=w602:dbl)
                      n405 = Square(x=w603) -> (x^2=w601:dbl)
                      n406 = Add(x=w602, y=w601) -> (x+y=w600:dbl)
                      n407 = Square(x=w593) -> (x^2=w592:dbl)
                      n408 = Square(x=w584) -> (x^2=w591:dbl)
                      n409 = global read "G_SEN.vi" "vision lane width"() -> (w597:dbl)
                      n410 = Subtract(x=w591, y=w592) -> (x-y=w542:dbl)
                      n411 = Square Root(x=w600) -> (sqrt(x)=w599:dbl)
                      n412 = Multiply(x=0.5, y=w525) -> (x*y=w522:dbl)
                      n413 = Subtract(x=w541, y=w599) -> (x-y=w598:dbl)
                      n414 = Max & Min(x=w542, y=w541) -> (max(x,y)=w540:dbl)  [unwired: 1 out]
                      n415 = global read "G_SEN.vi" "vision lane width"() -> (w589:dbl)
                      n416 = Compound Arithmetic op=ADD(w598, w531, w597) -> (w596:dbl)
                      n417 = Square Root(x=w540) -> (sqrt(x)=w590:dbl)
                      n418 = Add(x=w530, y=0.1) -> (x+y=w527:dbl)
                      n419 = Subtract(x=w584, y=w590) -> (x-y=w523:dbl)
                      n420 = Multiply(x=w596, y=0.5) -> (x*y=w528:dbl)
                      n421 = Max & Min(x=w528, y=w527) -> (max(x,y)=w526:dbl)  [unwired: 1 out]
                      n422 = Compound Arithmetic op=ADD(w523, w589) -> (w587:dbl)
                      n423 = Compound Arithmetic op=ADD(0.1 ("value"), w522, w523) -> (w519:dbl)
                      n424 = Multiply(x=w587, y=0.5) -> (x*y=w520:dbl)
                      n425 = Max & Min(x=w519, y=w520) -> (max(x,y)=w518:dbl)  [unwired: 1 out]
                      n426 = case shown="True" w580 {
                        tunnel: w582 -> [w614 w632]
                        tunnel: w581 -> [w613 _]
                        tunnel: w526 -> [w612 w635]
                        tunnel: [w611 w627] -> w579
                        tunnel: w518 -> [w610 w637]
                        frame False {
                          n427 = case shown="1" w614 {
                            tunnel: w613 -> [w619 w626]
                            tunnel: w612 -> [w616 w624]
                            tunnel: [w615 w620] -> w611
                            tunnel: w610 -> [w617 w623]
                            frame 0, Default {
                              n428 = Less Than 0?(x=w619) -> (x < 0?=w618:bool)
                              n429 = Select(t=w617, s=w618, f=w616) -> (s? t:f=w615:dbl)
                            }
                            frame 1 {
                              n430 = Greater Than 0?(x=w626) -> (x > 0?=w625:bool)
                              n431 = global read "G_SEN.vi" "vision lane width"() -> (w622:dbl)
                              n432 = Select(t=w623, s=w625, f=w624) -> (s? t:f=w621:dbl)
                              n433 = Subtract(x=w622, y=w621) -> (x-y=w620:dbl)
                            }
                          }
                        }
                        frame True {
                          n434 = Equal To 0?(x=w632) -> (x = 0?=w631:bool)
                          n435 = global read "G_SEN.vi" "vision lane width"() -> (w638:dbl)
                          n436 = Subtract(x=w638, y=w637) -> (x-y=w636:dbl)
                          n437 = global read "G_SEN.vi" "vision lane width"() -> (w630:dbl)
                          n438 = Add(x=w636, y=w635) -> (x+y=w633:dbl)
                          n439 = Multiply(x=w633, y=0.5) -> (x*y=w629:dbl)
                          n440 = Subtract(x=w630, y=w629) -> (x-y=w628:dbl)
                          n441 = Select(t=w629, s=w631, f=w628) -> (s? t:f=w627:dbl)
                        }
                      }
                      n442 = global read "G_SEN.vi" "vision lane width"() -> (w578:dbl)
                      n443 = local read "Coeff right"() -> (w564:dbl[])
                      n444 = local read "Coeff left"() -> (w551:dbl[])
                      n445 = global read "G_SEN.vi" "vision lane width"() -> (w562:dbl)
                      n446 = global read "G_SEN.vi" "vision lane width"() -> (w553:dbl)
                      n447 = Divide(x=w579, y=w578) -> (x/y=w538:dbl)
                      n448 = local read "poly"() -> (w569:i32)
                      n449 = local read "poly"() -> (w547:i32)
                      n450 = Increment(x=w569) -> (x+1=w568:i32)
                      n451 = Increment(x=w547) -> (x+1=w548:i32)
                      n452 = Index Array(array=w564, index #1=0 ("index")) -> (element #1=w563:dbl, element #2=w544:dbl)  [unwired: 1 in]
                      n453 = Index Array(array=w551, index #1=0 ("index")) -> (element #1=w552:dbl, element #2=w543:dbl)  [unwired: 1 in]
                      n454 = Subtract(x=0.5, y=w538) -> (x-y=w535:dbl)
                      n455 = local read "Coeff right"() -> (w557:dbl[])
                      n456 = Subtract(x=w563, y=w562) -> (x-y=w561:dbl)
                      n457 = Add(x=w552, y=w553) -> (x+y=w554:dbl)
                      n458 = Initialize Array(0.0 ("element"), w568) -> (w567:dbl[])
                      n459 = Initialize Array(0.0 ("element"), w548) -> (w549:dbl[])
                      n460 = local read "Coeff left"() -> (w572:dbl[])
                      n461 = Multiply(x=w535, y="gain") -> (x*y=w534:dbl)
                      n462 = Empty Array?(array=w557) -> (empty?=w559:bool)
                      n463 = Empty Array?(array=w572) -> (empty?=w573:bool)
                      n464 = Replace Array Subset(array=w567, new element #1=w561, index #1=0 ("index"), new element #2=w544) -> (w566:dbl[])  [unwired: 1 in]
                      n465 = Replace Array Subset(array=w549, new element #1=w554, index #1=0 ("index"), new element #2=w543) -> (w545:dbl[])  [unwired: 1 in]
                      n466 = Not(x=w559) -> (.not. x?=w558:bool)
                      n467 = Subtract(x=0.5 ("y"), y=w534) -> (x-y=w536:dbl)
                      n468 = Select(t=w566, s=w573, f=w572) -> (s? t:f=w571:dbl[])
                      n469 = Select(t=w557, s=w558, f=w545) -> (s? t:f=w556:dbl[])
                      n470 = Decrement(x=w536) -> (x-1=w577:dbl)
                      n471 = Multiply(x=w571, y=w536) -> (x*y=w575:dbl[])
                      n472 = Multiply(x=w577, y=w556) -> (x*y=w576:dbl[])
                      n473 = Subtract(x=w575, y=w576) -> (x-y=w574:dbl[])
                      n474 = global write "G_SEN.vi" "Lane_C_M"(w574) -> ()
                    }
                  }
                }
              }
              n475 = Subtract(x=0.5, y=w322) -> (x-y=w324:dbl)
              n476 = Multiply(x=w324, y=2.0) -> (x*y=→"ratio(-1:left1:right)":dbl)
            }
            frame #2 {
              n477 = global read "G_SEN.vi" "Lane_C_M"() -> (w639:dbl[])
              "Lane_C_M" <- w639
              n478 = Index Array(array=w639, index=0) -> (element=w641:dbl)
              n479 = Not A Number/Path/Refnum?(number/path/refnum=w641) -> (NaN/Path/Refnum?=w642:bool)
              n480 = case shown="True" w642 {
                selector: w642 -> [_ w643]
                frame False {
                }
                frame True {
                  "NaN/Path/Refnum?" <- w643
                }
              }
            }
          }
        }
        frame #2 {
          n481 = flat-sequence {
            frame #0 {
              n482 = global read "G_ALL.vi" "dist"() -> (→"map_dist":dbl[])
              n483 = global read "G_SEN.vi" "Lane_C_M"() -> (w656:dbl[])
              n484 = local read "y_end"() -> (w655:dbl[])
              n485 = global read "G_ALL.vi" "map_track 2"() -> (→"map_track":dbl[][])
              n486 = call-poly <vilib>:"Polynomial Evaluation.vi"("P(x)"=w656, "A"=w655) -> ("P(A)"=w654:dbl[])  [unwired: 1 out]
              n487 = Build Array(w654, w655) -> (w657:dbl[][])
              n488 = Transpose 2D Array(2D array=w657) -> (transposed array=w644:dbl[][])
              "lane_track" <- w644
              n489 = Delete From Array(array=w644, index (row)=0 ("index")) -> (deleted portion=w647:dbl[], array with subset deleted=w648:dbl[][])  [unwired: 2 in]
              n490 = for {
                tunnel: w648 -> [w658] mode=indexing
                shift-right: [w658] -> _
                shift-left: w647 -> [w665]
                shift-right: [w659] -> _
                shift-left: 0.0 -> [w660]
                tunnel: [w659] -> w650 mode=indexing
                n491 = Subtract(x=w658, y=w665) -> (x-y=w664:dbl[])
                n492 = Square(x=w664) -> (x^2=w663:dbl[])
                n493 = Add Array Elements(numeric array=w663) -> (sum=w662:dbl)
                n494 = Square Root(x=w662) -> (sqrt(x)=w661:dbl)
                n495 = Add(x=w661, y=w660) -> (x+y=w659:dbl)
              }
              n496 = Build Array (concatenate)(0.0, w650) -> (→"lane dist":dbl[])
            }
            frame #1 {
              n497 = local read "map_track"() -> (w693:dbl[][])
              n498 = local read "lane_track"() -> (w696:dbl[][])
              n499 = Index Array(array=w693, index (col) #1=0 ("disabled index (col)")) -> (element #1=w692:dbl[], element #2=w709:dbl[])  [unwired: 3 in]
              n500 = Index Array(array=w696, index (col) #1=0 ("disabled index (col)")) -> (element #1=w691:dbl[], element #2=w694:dbl[])  [unwired: 3 in]
              n501 = Array Size(array=w692) -> (size(s)=w698:i32)
              n502 = Array Size(array=w691) -> (size(s)=w695:i32)
              n503 = local read "map_dist"() -> (w690:dbl[])
              n504 = local read "lane dist"() -> (w689:dbl[])
              n505 = Decrement(x=w698) -> (x-1=w712:i32)
              n506 = Decrement(x=w695) -> (x-1=w704:i32)
              n507 = for {
                tunnel: w692 -> [w964]
                tunnel: w709 -> [w963]
                tunnel: [w979] -> w711 mode=indexing
                tunnel: w712 -> [w978]
                tunnel: [w958] -> w710 mode=indexing
                tunnel: [w960] -> w703
                tunnel: 5.0 ("x") -> [w965]
                tunnel: w690 -> [w955] mode=indexing
                tunnel: w690 -> [w957]
                i -> [w960]
                stop <- w977 stop-if-true
                n508 = Add(x=w955, y=w965) -> (x+y=w966:dbl)
                n509 = Subtract(x=w955, y=w965) -> (x-y=w956:dbl)
                n510 = Index Array(array=w964, index=w960) -> (element=w1005:dbl)
                n511 = Index Array(array=w963, index=w960) -> (element=w1004:dbl)
                n512 = Threshold 1D Array(2:w956, 3:w957) -> (0:w1010:dbl)  [unwired: 1 in]
                n513 = Threshold 1D Array(1:w960, 2:w966, 3:w957) -> (0:w961:dbl)
                n514 = Greater Or Equal?(x=w961, y=w978) -> (x >= y?=w977:bool)
                n515 = Interpolate 1D Array(1:w961, 2:w964) -> (0:w1008:dbl)
                n516 = Interpolate 1D Array(1:w961, 2:w963) -> (0:w1007:dbl)
                n517 = Interpolate 1D Array(1:w1010, 2:w964) -> (0:w959:dbl)
                n518 = Interpolate 1D Array(1:w1010, 2:w963) -> (0:w1009:dbl)
                n519 = Build Array(w1005, w1004) -> (w973:dbl[])
                n520 = Build Array(w1008, w1007) -> (w1006:dbl[])
                n521 = Build Array(w959, w1009) -> (w962:dbl[])
                n522 = Build Array(w973, w962, w1006) -> (w976:dbl[][])
                n523 = Build Array(w962, w962, w962) -> (w975:dbl[][])
                n524 = Subtract(x=w976, y=w975) -> (x-y=w974:dbl[][])
                n525 = Transpose 2D Array(2D array=w974) -> (transposed array=w985:dbl[][])
                n526 = Index Array(array=w974, index (col) #1=0 ("disabled index (col)")) -> (element #1=w981:dbl[], element #2=w982:dbl[])  [unwired: 3 in]
                n527 = Square(x=w981) -> (x^2=w983:dbl[])
                n528 = Square(x=w982) -> (x^2=w984:dbl[])
                n529 = Add(x=w983, y=w984) -> (x+y=w986:dbl[])
                n530 = Build Array (concatenate)(w985, dbl[] [1.0, 1.0, 1.0] ("initialized array")) -> (w995:dbl[][])
                n531 = Negate(x=w986) -> (-x=w987:dbl[])
                n532 = Transpose 2D Array(2D array=w995) -> (transposed array=w996:dbl[][])
                n533 = call-poly <vilib>:"Solve Linear Equations.vi"("Known Vector"=w987, "Input Matrix"=w996) -> ("Solution Vector"=w988:dbl[])  [unwired: 1 in, 1 out]
                n534 = Index Array(array=w988, index #1=0 ("index")) -> (element #1=w958:dbl, element #2=w990:dbl, element #3=w993:dbl)  [unwired: 2 in]
                n535 = Square(x=w958) -> (x^2=w991:dbl)
                n536 = Square(x=w990) -> (x^2=w992:dbl)
                n537 = Add(x=w991, y=w992) -> (x+y=w972:dbl)
                n538 = Multiply(x=w993, y=1.0) -> (x*y=w994:dbl)
                n539 = Square Root(x=w972) -> (sqrt(x)=w971:dbl)
                n540 = Multiply(x=0.25, y=w972) -> (x*y=w1001:dbl)
                n541 = Subtract(x=w1001, y=w994) -> (x-y=w997:dbl)
                n542 = Greater?(x=w971, y=1.0) -> (0:w968:bool)
                n543 = Greater Than 0?(x=w997) -> (x > 0?=w969:bool)
                n544 = And(x=w969, y=w968) -> (x .and. y?=w967:bool)
                n545 = Square Root(x=w997) -> (sqrt(x)=w1003:dbl)
                n546 = Select(t=w1003, s=w967, f=inf) -> (s? t:f=w979:dbl)
              }
              n547 = for {
                tunnel: w691 -> [w909]
                tunnel: w694 -> [w908]
                tunnel: [w924] -> w705 mode=indexing
                tunnel: w704 -> [w923]
                tunnel: [w902] -> w706 mode=indexing
                tunnel: [w905] -> w702
                tunnel: 5.0 ("x") -> [w910]
                tunnel: w689 -> [w900] mode=indexing
                tunnel: w689 -> [w901]
                tunnel: [w899] -> _ mode=indexing
                i -> [w905]
                stop <- w922 stop-if-true
                n548 = Add(x=w900, y=w910) -> (x+y=w911:dbl)
                n549 = Subtract(x=w900, y=w910) -> (x-y=w904:dbl)
                n550 = Index Array(array=w909, index=w905) -> (element=w950:dbl)
                n551 = Index Array(array=w908, index=w905) -> (element=w949:dbl)
                n552 = Threshold 1D Array(1:w905, 2:w911, 3:w901) -> (0:w906:dbl)
                n553 = Threshold 1D Array(2:w904, 3:w901) -> (0:w899:dbl)  [unwired: 1 in]
                n554 = Greater Or Equal?(x=w906, y=w923) -> (x >= y?=w922:bool)
                n555 = Interpolate 1D Array(1:w906, 2:w909) -> (0:w953:dbl)
                n556 = Interpolate 1D Array(1:w906, 2:w908) -> (0:w952:dbl)
                n557 = Interpolate 1D Array(1:w899, 2:w909) -> (0:w903:dbl)
                n558 = Interpolate 1D Array(1:w899, 2:w908) -> (0:w954:dbl)
                n559 = Build Array(w950, w949) -> (w918:dbl[])
                n560 = Build Array(w953, w952) -> (w951:dbl[])
                n561 = Build Array(w903, w954) -> (w907:dbl[])
                n562 = Build Array(w918, w907, w951) -> (w921:dbl[][])
                n563 = Build Array(w907, w907, w907) -> (w920:dbl[][])
                n564 = Subtract(x=w921, y=w920) -> (x-y=w919:dbl[][])
                n565 = Transpose 2D Array(2D array=w919) -> (transposed array=w930:dbl[][])
                n566 = Index Array(array=w919, index (col) #1=0 ("disabled index (col)")) -> (element #1=w926:dbl[], element #2=w927:dbl[])  [unwired: 3 in]
                n567 = Square(x=w926) -> (x^2=w928:dbl[])
                n568 = Square(x=w927) -> (x^2=w929:dbl[])
                n569 = Add(x=w928, y=w929) -> (x+y=w931:dbl[])
                n570 = Build Array (concatenate)(w930, dbl[] [1.0, 1.0, 1.0] ("initialized array")) -> (w940:dbl[][])
                n571 = Negate(x=w931) -> (-x=w932:dbl[])
                n572 = Transpose 2D Array(2D array=w940) -> (transposed array=w941:dbl[][])
                n573 = call-poly <vilib>:"Solve Linear Equations.vi"("Known Vector"=w932, "Input Matrix"=w941) -> ("Solution Vector"=w933:dbl[])  [unwired: 1 in, 1 out]
                n574 = Index Array(array=w933, index #1=0 ("index")) -> (element #1=w902:dbl, element #2=w935:dbl, element #3=w938:dbl)  [unwired: 2 in]
                n575 = Square(x=w902) -> (x^2=w936:dbl)
                n576 = Square(x=w935) -> (x^2=w937:dbl)
                n577 = Add(x=w936, y=w937) -> (x+y=w917:dbl)
                n578 = Multiply(x=w938, y=1.0) -> (x*y=w939:dbl)
                n579 = Square Root(x=w917) -> (sqrt(x)=w916:dbl)
                n580 = Multiply(x=0.25, y=w917) -> (x*y=w946:dbl)
                n581 = Subtract(x=w946, y=w939) -> (x-y=w942:dbl)
                n582 = Greater?(x=w916, y=1.0) -> (0:w913:bool)
                n583 = Greater Than 0?(x=w942) -> (x > 0?=w914:bool)
                n584 = And(x=w914, y=w913) -> (x .and. y?=w912:bool)
                n585 = Square Root(x=w942) -> (sqrt(x)=w948:dbl)
                n586 = Select(t=w948, s=w912, f=inf) -> (s? t:f=w924:dbl)
              }
              n587 = Array Subset(array=w710, index=1, length=w703) -> (w688:dbl[])
              n588 = Array Subset(array=w711, index=1, length=w703) -> (w687:dbl[])
              n589 = Array Subset(array=w706, index=1, length=w702) -> (w681:dbl[])
              n590 = Array Subset(array=w705, index=1, length=w702) -> (w682:dbl[])
              n591 = Sign(1:w688) -> (0:w685:dbl[])
              n592 = Sign(1:w681) -> (0:w684:dbl[])
              n593 = Multiply(x=w685, y=w687) -> (x*y=w686:dbl[])
              n594 = Multiply(x=w684, y=w682) -> (x*y=w683:dbl[])
              n595 = Reciprocal(x=w686) -> (1/x=w680:dbl[])
              n596 = Reciprocal(x=w683) -> (1/x=w674:dbl[])
              n597 = flat-sequence {
                tunnel: w680 -> [w825]
                tunnel: [w823] -> w676
                tunnel: [w825] -> w675
                tunnel: w674 -> [w822]
                tunnel: [w864] -> w679
                tunnel: [w835] -> w678
                tunnel: [w834] -> w677
                tunnel: w676 -> [w836]
                tunnel: w675 -> [w837]
                tunnel: [w836] -> w673
                frame #0 {
                  n598 = local read "lane dist"() -> (w827:dbl[])
                  n599 = Array Size(array=w822) -> (size(s)=w828:i32)
                  n600 = Array Subset(array=w827, index=1, length=w828) -> (w824:dbl[])
                  n601 = call <vilib>:"General Polynomial Fit Coefficients.vi"("Y"=w822, "polynomial order"=3, "X"=w824) -> ("Polynomial Coefficients"=w823:dbl[])  [unwired: 11 in, 1 out]
                  n602 = call-poly <vilib>:"Polynomial Evaluation.vi"("P(x)"=w823, "A"=w824) -> ("P(A)"=w821:dbl[])  [unwired: 1 out]
                  n603 = Build Array(w822, w821) -> (→"range 2":dbl[][])
                  "range" <- w825
                }
                frame #1 {
                  n604 = Array Size(array=w837) -> (size(s)=w846:i32)
                  n605 = call-poly <vilib>:"nth Derivative of Polynomial.vi"("order"=1, "P(x)"=w836) -> ("Nth Derivative of P(x)"=w862:dbl[])  [unwired: 8 in, 1 out]
                  n606 = local read "map_dist"() -> (w847:dbl[])
                  n607 = call-poly <vilib>:"Polynomial Roots.vi"("P(x)"=w862) -> ("Roots"=w861:cdb[])  [unwired: 9 in, 1 out]
                  n608 = Array Subset(array=w847, index=1, length=w846) -> (w840:dbl[])
                  n609 = Complex To Re/Im(x + iy=w861) -> (x=w852:dbl[], y=w860:dbl[])
                  n610 = Equal To 0?(x=w860) -> (x = 0?=w850:bool[])
                  n611 = In Range and Coerce(upper limit=8.0, x=w840, lower limit=-6.0) -> (In Range?=w842:bool[])  [unwired: 1 out]
                  n612 = In Range and Coerce(upper limit=10.0, x=w852, lower limit=0.0) -> (In Range?=w851:bool[])  [unwired: 1 out]
                  n613 = Boolean To (0,1)(Boolean=w842) -> (0, 1=w841:i16[])
                  n614 = And(x=w850, y=w851) -> (x .and. y?=w849:bool[])
                  n615 = Add Array Elements(numeric array=w841) -> (sum=w838:i16)
                  n616 = Boolean To (0,1)(Boolean=w849) -> (0, 1=w856:i16[])
                  n617 = Array Max & Min(array=w841) -> (max index (indices)=w839:i32)  [unwired: 3 out]
                  n618 = Build Cluster Array(w849, w852) -> (w859:cluster{bool, dbl}[])
                  n619 = Add Array Elements(numeric array=w856) -> (sum=w855:i16)
                  n620 = Array Subset(array=w837, index=w839, length=w838) -> (w830:dbl[])
                  n621 = Array Subset(array=w840, index=w839, length=w838) -> (w833:dbl[])
                  n622 = Sort 1D Array(array=w859) -> (sorted array=w858:cluster{bool, dbl}[])
                  n623 = Reverse 1D Array(array=w858) -> (reversed array=w857:cluster{bool, dbl}[])
                  n624 = call <vilib>:"General Polynomial Fit Coefficients.vi"("Y"=w830, "polynomial order"=5, "X"=w833) -> ("Polynomial Coefficients"=w834:dbl[])  [unwired: 11 in, 1 out]
                  n625 = for {
                    N: w855 -> [_]
                    tunnel: w857 -> [w866] mode=indexing
                    tunnel: [w865] -> w835 mode=indexing
                    n626 = Unbundle(w866) -> (w865:dbl)  [unwired: 1 out]
                  }
                  n627 = call-poly <vilib>:"Polynomial Evaluation.vi"("P(x)"=w834, "A"=w833) -> ("P(A)"=w832:dbl[])  [unwired: 1 out]
                  n628 = Build Array(w830, w832) -> (→"range 3":dbl[][])
                  n629 = Empty Array?(array=w835) -> (empty?=w864:bool)
                }
              }
              n630 = case shown="False" w679 {
                tunnel: w673 -> [w871 w880]
                tunnel: w678 -> [w873 _]
                tunnel: [w869 w878] -> w672
                tunnel: [w867 w876] -> w671
                tunnel: [_ w874] -> w666
                frame False {
                  n631 = Array Max & Min(array=w873) -> (min value=w869:dbl)  [unwired: 3 out]
                  n632 = call-poly <vilib>:"nth Derivative of Polynomial.vi"("order"=2, "P(x)"=w871) -> ("Nth Derivative of P(x)"=w870:dbl[])  [unwired: 8 in, 1 out]
                  n633 = call-poly <vilib>:"Polynomial Evaluation.vi"("P(x)"=w870, "a"=w869) -> ("P(a)"=w868:dbl)  [unwired: 1 out]
                  n634 = Sign(1:w868) -> (0:w867:dbl)
                }
                frame True {
                  n635 = call-poly <vilib>:"Polynomial Roots.vi"("P(x)"=w880) -> ("Roots"=w888:cdb[])  [unwired: 9 in, 1 out]
                  n636 = Complex To Re/Im(x + iy=w888) -> (x=w885:dbl[], y=w889:dbl[])
                  n637 = Equal To 0?(x=w889) -> (x = 0?=w883:bool[])
                  n638 = In Range and Coerce(upper limit=10.0, x=w885, lower limit=0.0) -> (In Range?=w882:bool[])  [unwired: 1 out]
                  n639 = And(x=w883, y=w882) -> (x .and. y?=w884:bool[])
                  n640 = Boolean To (0,1)(Boolean=w884) -> (0, 1=w893:i16[])
                  n641 = Build Cluster Array(w884, w885) -> (w890:cluster{bool, dbl}[])
                  n642 = Add Array Elements(numeric array=w893) -> (sum=w894:i16)
                  n643 = Sort 1D Array(array=w890) -> (sorted array=w891:cluster{bool, dbl}[])
                  n644 = Reverse 1D Array(array=w891) -> (reversed array=w892:cluster{bool, dbl}[])
                  n645 = for {
                    N: w894 -> [_]
                    tunnel: w892 -> [w896] mode=indexing
                    tunnel: [w895] -> w875 mode=indexing
                    n646 = Unbundle(w896) -> (w895:dbl)  [unwired: 1 out]
                  }
                  n647 = call-poly <vilib>:"nth Derivative of Polynomial.vi"("order"=1, "P(x)"=w880) -> ("Nth Derivative of P(x)"=w879:dbl[])  [unwired: 8 in, 1 out]
                  n648 = Empty Array?(array=w875) -> (empty?=w874:bool)
                  n649 = Array Max & Min(array=w875) -> (min value=w878:dbl)  [unwired: 3 out]
                  n650 = call-poly <vilib>:"Polynomial Evaluation.vi"("P(x)"=w879, "a"=w878) -> ("P(a)"=w877:dbl)  [unwired: 1 out]
                  n651 = Sign(1:w877) -> (0:w876:dbl)
                }
              }
              n652 = case shown="False" w666 {
                tunnel: [w721 _] -> w701
                tunnel: [w720 _] -> w700
                tunnel: w679 -> [w718 _]
                tunnel: w677 -> [w717 _]
                tunnel: w672 -> [w716 _]
                tunnel: w671 -> [w715 _]
                frame False {
                  n653 = case shown="False" w718 {
                    tunnel: w717 -> [w774 w803]
                    tunnel: [w767 w795] -> w719
                    tunnel: w715 -> [w766 w799]
                    tunnel: [w764 w793] -> w714
                    frame False {
                      n654 = call-poly <vilib>:"nth Derivative of Polynomial.vi"("order"=1, "P(x)"=w774) -> ("Nth Derivative of P(x)"=w777:dbl[])  [unwired: 8 in, 1 out]
                      n655 = call-poly <vilib>:"Polynomial Roots.vi"("P(x)"=w777) -> ("Roots"=w778:cdb[])  [unwired: 9 in, 1 out]
                      n656 = Complex To Re/Im(x + iy=w778) -> (x=w787:dbl[], y=w779:dbl[])
                      n657 = Equal To 0?(x=w779) -> (x = 0?=w789:bool[])
                      n658 = In Range and Coerce(upper limit=8.0, x=w787, lower limit=-6.0) -> (In Range?=w788:bool[])  [unwired: 1 out]
                      n659 = And(x=w789, y=w788) -> (x .and. y?=w790:bool[])
                      n660 = Boolean To (0,1)(Boolean=w790) -> (0, 1=w783:i16[])
                      n661 = Build Cluster Array(w790, w787) -> (w780:cluster{bool, dbl}[])
                      n662 = Add Array Elements(numeric array=w783) -> (sum=w784:i16)
                      n663 = Sort 1D Array(array=w780) -> (sorted array=w781:cluster{bool, dbl}[])
                      n664 = Reverse 1D Array(array=w781) -> (reversed array=w782:cluster{bool, dbl}[])
                      n665 = for {
                        N: w784 -> [_]
                        tunnel: w782 -> [w792] mode=indexing
                        tunnel: [w791] -> w765 mode=indexing
                        n666 = Unbundle(w792) -> (w791:dbl)  [unwired: 1 out]
                      }
                      n667 = call-poly <vilib>:"nth Derivative of Polynomial.vi"("order"=2, "P(x)"=w774) -> ("Nth Derivative of P(x)"=w773:dbl[])  [unwired: 8 in, 1 out]
                      n668 = Sort 1D Array(array=w765) -> (sorted array=w764:dbl[])
                      n669 = call-poly <vilib>:"Polynomial Evaluation.vi"("P(x)"=w773, "A"=w764) -> ("P(A)"=w772:dbl[])  [unwired: 1 out]
                      n670 = Sign(1:w772) -> (0:w771:dbl[])
                      n671 = Equal?(x=w771, y=w766) -> (x = y?=w770:bool[])
                      n672 = Boolean To (0,1)(Boolean=w770) -> (0, 1=w769:i16[])
                      n673 = Array Max & Min(array=w769) -> (max index (indices)=w768:i32)  [unwired: 3 out]
                      n674 = Index Array(array=w764, index=w768) -> (element=w767:dbl)
                    }
                    frame True {
                      n675 = call-poly <vilib>:"Polynomial Roots.vi"("P(x)"=w803) -> ("Roots"=w811:cdb[])  [unwired: 9 in, 1 out]
                      n676 = Complex To Re/Im(x + iy=w811) -> (x=w808:dbl[], y=w812:dbl[])
                      n677 = Equal To 0?(x=w812) -> (x = 0?=w806:bool[])
                      n678 = In Range and Coerce(upper limit=8.0, x=w808, lower limit=-6.0) -> (In Range?=w805:bool[])  [unwired: 1 out]
                      n679 = And(x=w806, y=w805) -> (x .and. y?=w807:bool[])
                      n680 = Boolean To (0,1)(Boolean=w807) -> (0, 1=w816:i16[])
                      n681 = Build Cluster Array(w807, w808) -> (w813:cluster{bool, dbl}[])
                      n682 = Add Array Elements(numeric array=w816) -> (sum=w817:i16)
                      n683 = Sort 1D Array(array=w813) -> (sorted array=w814:cluster{bool, dbl}[])
                      n684 = Reverse 1D Array(array=w814) -> (reversed array=w815:cluster{bool, dbl}[])
                      n685 = for {
                        N: w817 -> [_]
                        tunnel: w815 -> [w819] mode=indexing
                        tunnel: [w818] -> w794 mode=indexing
                        n686 = Unbundle(w819) -> (w818:dbl)  [unwired: 1 out]
                      }
                      n687 = call-poly <vilib>:"nth Derivative of Polynomial.vi"("order"=1, "P(x)"=w803) -> ("Nth Derivative of P(x)"=w802:dbl[])  [unwired: 8 in, 1 out]
                      n688 = Sort 1D Array(array=w794) -> (sorted array=w793:dbl[])
                      n689 = call-poly <vilib>:"Polynomial Evaluation.vi"("P(x)"=w802, "A"=w793) -> ("P(A)"=w801:dbl[])  [unwired: 1 out]
                      n690 = Sign(1:w801) -> (0:w800:dbl[])
                      n691 = Equal?(x=w799, y=w800) -> (x = y?=w796:bool[])
                      n692 = Boolean To (0,1)(Boolean=w796) -> (0, 1=w798:i16[])
                      n693 = Array Max & Min(array=w798) -> (max index (indices)=w797:i32)  [unwired: 3 out]
                      n694 = Index Array(array=w793, index=w797) -> (element=w795:dbl)
                    }
                  }
                  n695 = Empty Array?(array=w714) -> (empty?=w713:bool)
                  n696 = case shown="False" w713 {
                    tunnel: [w743 _] -> w721
                    tunnel: [w742 _] -> w720
                    tunnel: w719 -> [w729 _]
                    tunnel: w716 -> [w728 _]
                    frame False {
                      n697 = disable-structure shown="Enabled" {
                        disable-tunnel: [w758 35.0] -> w734
                        disable-tunnel: w728 -> [w762 _]
                        frame Enabled {
                          n698 = local read "lane dist"() -> (w761:dbl[])
                          n699 = Array Subset(array=w761, index=1) -> (w759:dbl[])  [unwired: 1 in]
                          n700 = Threshold 1D Array(2:w762, 3:w759) -> (0:w758:dbl)  [unwired: 1 in]
                          "fractional index or x 2" <- w758
                        }
                        frame Disabled {
                        }
                      }
                      n701 = disable-structure shown="Enabled" {
                        disable-tunnel: [w756 0.0] -> w738
                        disable-tunnel: w729 -> [w752 _]
                        frame Enabled {
                          n702 = local read "map_dist"() -> (w754:dbl[])
                          n703 = Add(x=w752, y="y 2") -> (x+y=w751:dbl)
                          n704 = Array Subset(array=w754, index=1) -> (w753:dbl[])  [unwired: 1 in]
                          n705 = Threshold 1D Array(2:w751, 3:w753) -> (0:w756:dbl)  [unwired: 1 in]
                          "fractional index or x" <- w756
                        }
                        frame Disabled {
                        }
                      }
                      n706 = local read "lane_track"() -> (w723:dbl[][])
                      n707 = Array Subset(array=w723, index (row)=1 ("index")) -> (w722:dbl[][])  [unwired: 3 in]
                      n708 = local read "map_track"() -> (w727:dbl[][])
                      n709 = Index Array(array=w722, index (col) #1=0 ("disabled index (col)")) -> (element #1=w731:dbl[], element #2=w730:dbl[])  [unwired: 3 in]
                      n710 = disable-structure shown="Enabled" {
                        disable-tunnel: [w749 _] -> w737
                        disable-tunnel: w734 -> [w748 _]
                        disable-tunnel: w731 -> [w747 _]
                        frame Enabled {
                          n711 = Interpolate 1D Array(1:w748, 2:w747) -> (0:w749:dbl)
                        }
                        frame Disabled {
                        }
                      }
                      n712 = disable-structure shown="Enabled" {
                        disable-tunnel: w734 -> [w746 _]
                        disable-tunnel: [w745 _] -> w733
                        disable-tunnel: w730 -> [w744 _]
                        frame Enabled {
                          n713 = Interpolate 1D Array(1:w746, 2:w744) -> (0:w745:dbl)
                        }
                        frame Disabled {
                        }
                      }
                      n714 = Array Subset(array=w727, index (row)=1 ("index")) -> (w726:dbl[][])  [unwired: 3 in]
                      n715 = Index Array(array=w726, index (col) #1=0 ("disabled index (col)")) -> (element #1=w740:dbl[], element #2=w739:dbl[])  [unwired: 3 in]
                      n716 = Interpolate 1D Array(1:w738, 2:w740) -> (0:w736:dbl)
                      n717 = Interpolate 1D Array(1:w738, 2:w739) -> (0:w735:dbl)
                      n718 = Subtract(x=w737, y=w736) -> (x-y=w743:dbl)
                      n719 = Subtract(x=w733, y=w735) -> (x-y=w742:dbl)
                    }
                    frame True {
                    }
                  }
                }
                frame True {
                }
              }
              n720 = disable-structure shown="Enabled" {
                disable-tunnel: w701 -> [w898 _]
                disable-tunnel: w700 -> [w897 _]
                frame Enabled {
                  "x_shift" <- w898
                  "y_shift" <- w897
                }
                frame Disabled {
                }
              }
            }
          }
        }
        frame #3 {
          n721 = local read "w"() -> (→"Waveform Graph":dbl[])
          n722 = local read "w"() -> (w1100:dbl[])
          n723 = local read "w"() -> (w1080:dbl[])
          n724 = Equal?(x=w1100, y=-1.0) -> (x = y?=w1098:bool[])
          n725 = Equal?(x=w1080, y=1.0) -> (x = y?=w1082:bool[])
          n726 = local read "x"() -> (w1097:dbl[])
          n727 = local read "y"() -> (w1096:dbl[])
          n728 = local read "x"() -> (w1083:dbl[])
          n729 = local read "y"() -> (w1084:dbl[])
          n730 = Build Cluster Array(w1098, w1097, w1096) -> (w1095:cluster{bool, dbl, dbl}[])
          n731 = Build Cluster Array(w1082, w1083, w1084) -> (w1085:cluster{bool, dbl, dbl}[])
          n732 = Sort 1D Array(array=w1095) -> (sorted array=w1094:cluster{bool, dbl, dbl}[])
          n733 = Sort 1D Array(array=w1085) -> (sorted array=w1086:cluster{bool, dbl, dbl}[])
          n734 = Reverse 1D Array(array=w1094) -> (reversed array=w1093:cluster{bool, dbl, dbl}[])
          n735 = Reverse 1D Array(array=w1086) -> (reversed array=w1087:cluster{bool, dbl, dbl}[])
          n736 = for {
            tunnel: w1093 -> [w1114] mode=indexing
            tunnel: [w1112] -> w1092 mode=indexing
            tunnel: [w1111] -> w1073 mode=indexing
            tunnel: [w1110] -> w1091
            i -> [w1110]
            stop <- w1113 continue-if-true
            n737 = Unbundle(w1114) -> (w1113:bool, w1112:dbl, w1111:dbl)
          }
          n738 = for {
            tunnel: w1087 -> [w1109] mode=indexing
            tunnel: [w1107] -> w1088 mode=indexing
            tunnel: [w1106] -> w1069 mode=indexing
            tunnel: [w1105] -> w1089
            i -> [w1105]
            stop <- w1108 continue-if-true
            n739 = Unbundle(w1109) -> (w1108:bool, w1107:dbl, w1106:dbl)
          }
          n740 = Array Subset(array=w1092, index=0, length=w1091) -> (w1090:dbl[])
          n741 = Array Subset(array=w1088, index=0, length=w1089) -> (w1079:dbl[])
          n742 = Array Subset(array=w1073, index=0, length=w1091) -> (w1068:dbl[])
          n743 = Array Subset(array=w1069, index=0, length=w1089) -> (w1064:dbl[])
          n744 = call "Convert to Dynamic Data4"("Array"=w1090) -> ("Dynamic Data Type"=w1053:dynamicdata)  [unwired: 3 in]
          n745 = call "Convert to Dynamic Data6"("Array"=w1079) -> ("Dynamic Data Type"=w1051:dynamicdata)  [unwired: 3 in]
          n746 = call "Convert to Dynamic Data3"("Array"=w1068) -> ("Dynamic Data Type"=w1065:dynamicdata)  [unwired: 3 in]
          n747 = Array Max & Min(array=w1068) -> (max value=w1075:dbl, min value=w1074:dbl)  [unwired: 2 out]
          n748 = Array Max & Min(array=w1064) -> (max value=w1071:dbl, min value=w1072:dbl)  [unwired: 2 out]
          n749 = call "Convert to Dynamic Data8"("Array"=w1064) -> ("Dynamic Data Type"=w1063:dynamicdata)  [unwired: 3 in]
          n750 = Increment(x=w1075) -> (x+1=w1036:dbl)
          n751 = Decrement(x=w1074) -> (x-1=w1031:dbl)
          n752 = Increment(x=w1071) -> (x+1=w1035:dbl)
          n753 = Decrement(x=w1072) -> (x-1=w1030:dbl)
          n754 = global read "G_ALL.vi" "map_track 2"() -> (w1021:dbl[][])
          n755 = Add(x=w1036, y=w1035) -> (x+y=w1034:dbl)
          n756 = Add(x=w1031, y=w1030) -> (x+y=w1028:dbl)
          n757 = call-poly <vilib>:"Ramp Pattern.vi"("start"=w1031, "end"=w1036, "delta"=0.01) -> ("Ramp Pattern"=w1040:dbl[])  [unwired: 6 in, 2 out]
          n758 = call-poly <vilib>:"Ramp Pattern.vi"("start"=w1030, "end"=w1035, "delta"=0.01) -> ("Ramp Pattern"=w1039:dbl[])  [unwired: 6 in, 2 out]
          n759 = local read "Coeff right"() -> (w1038:dbl[])
          n760 = local read "Coeff stop"() -> (w1078:dbl[])
          n761 = local read "Coeff left"() -> (w1103:dbl[])
          n762 = Index Array(array=w1021, index (col) #1=0 ("disabled index (col)")) -> (element #1=w1014:dbl[], element #2=w1016:dbl[])  [unwired: 3 in]
          n763 = Multiply(x=w1034, y=0.5) -> (x*y=w1032:dbl)
          n764 = Multiply(x=w1028, y=0.5) -> (x*y=w1027:dbl)
          n765 = call-poly <vilib>:"Polynomial Evaluation.vi"("P(x)"=w1103, "A"=w1040) -> ("P(A)"=w1046:dbl[])  [unwired: 1 out]
          n766 = call-poly <vilib>:"Polynomial Evaluation.vi"("P(x)"=w1038, "A"=w1039) -> ("P(A)"=w1041:dbl[])  [unwired: 1 out]
          n767 = local read "y_shift"() -> (w1012:dbl)
          n768 = local read "x_shift"() -> (w1011:dbl)
          n769 = call "Convert to Dynamic Data7"("Array"=w1040) -> ("Dynamic Data Type"=w1050:dynamicdata)  [unwired: 3 in]
          n770 = call "Convert to Dynamic Data11"("Array"=w1039) -> ("Dynamic Data Type"=w1049:dynamicdata)  [unwired: 3 in]
          n771 = local read "y_end"() -> (w1077:dbl[])
          n772 = call-poly <vilib>:"Ramp Pattern.vi"("start"=w1027, "end"=w1032, "delta"=0.01) -> ("Ramp Pattern"=w1023:dbl[])  [unwired: 6 in, 2 out]
          n773 = global read "G_SEN.vi" "Lane_C_M"() -> (w1026:dbl[])
          n774 = Add(x=w1014, y=w1011) -> (x+y=w1013:dbl[])
          n775 = call-poly <vilib>:"Polynomial Evaluation.vi"("P(x)"=w1078, "A"=w1077) -> ("P(A)"=w1047:dbl[])  [unwired: 1 out]
          n776 = Add(x=w1016, y=w1012) -> (x+y=w1015:dbl[])
          n777 = Build Array(w1046, w1040) -> (w1045:dbl[][])
          n778 = Build Array(w1041, w1039) -> (w1042:dbl[][])
          n779 = call "Convert to Dynamic Data2"("Array"=w1046) -> ("Dynamic Data Type"=w1054:dynamicdata)  [unwired: 3 in]
          n780 = call "Convert to Dynamic Data5"("Array"=w1041) -> ("Dynamic Data Type"=w1052:dynamicdata)  [unwired: 3 in]
          n781 = local read "y"() -> (w1102:dbl[])
          n782 = local read "y_end"() -> (w1048:dbl[])
          n783 = call-poly <vilib>:"Polynomial Evaluation.vi"("P(x)"=w1026, "A"=w1023) -> ("P(A)"=w1025:dbl[])  [unwired: 1 out]
          n784 = Transpose 2D Array(2D array=w1045) -> (transposed array=w1044:dbl[][])
          n785 = Transpose 2D Array(2D array=w1042) -> (transposed array=w1043:dbl[][])
          n786 = call "Convert to Dynamic Data15"("Array"=w1013) -> ("Dynamic Data Type"=w1019:dynamicdata)  [unwired: 3 in]
          n787 = call "Convert to Dynamic Data14"("Array"=w1023) -> ("Dynamic Data Type"=w1022:dynamicdata)  [unwired: 3 in]
          n788 = call "Convert to Dynamic Data"("Array"=w1047) -> ("Dynamic Data Type"=w1059:dynamicdata)  [unwired: 3 in]
          n789 = call "Convert to Dynamic Data16"("Array"=w1015) -> ("Dynamic Data Type"=w1018:dynamicdata)  [unwired: 3 in]
          n790 = call "Convert to Dynamic Data10"("Array"=w1102) -> ("Dynamic Data Type"=w1061:dynamicdata)  [unwired: 3 in]
          n791 = local read "x"() -> (w1101:dbl[])
          n792 = global write "G_SEN.vi" "Lane_L_V"(w1044) -> ()
          n793 = call "Convert to Dynamic Data12"("Array"=w1048) -> ("Dynamic Data Type"=w1060:dynamicdata)  [unwired: 3 in]
          n794 = call "Convert to Dynamic Data13"("Array"=w1025) -> ("Dynamic Data Type"=w1024:dynamicdata)  [unwired: 3 in]
          n795 = Merge Signals(w1050, w1065, w1049, w1063, w1061, w1059, w1022, w1018) -> (w1066:dynamicdata)
          n796 = global write "G_SEN.vi" "Lane_R_V"(w1043) -> ()
          n797 = call "Convert to Dynamic Data9"("Array"=w1101) -> ("Dynamic Data Type"=w1062:dynamicdata)  [unwired: 3 in]
          n798 = Merge Signals(w1054, w1053, w1052, w1051, w1062, w1060, w1024, w1019) -> (w1067:dynamicdata)
          n799 = call "Build XY Graph"("Y Input"=w1066, "X Input"=w1067) -> ("XY Graph"=→"XY Graph 4":cluster{"X":dbl[], "Y":dbl[]}[])  [unwired: 8 in, 1 out]
        }
      }
    }
    frame True {
      w1116 = dbl[][] [] ("Lane_R_V")
      n800 = disable-structure shown="Enabled" {
        frame Enabled {
          w1122 = dbl[] [] ("Coeff left")
          n801 = local write "Coeff left"(w1122) -> ()
          n802 = local write "Coeff right"(w1122) -> ()
        }
        frame Disabled {
        }
      }
      n803 = call-poly <vilib>:"Ramp Pattern.vi"("start"=-4.0, "end"=6.0, "delta"=0.1) -> ("Ramp Pattern"=→"y_end":dbl[])  [unwired: 6 in, 2 out]
      n804 = global write "G_SEN.vi" "Lane_L_V"(w1116) -> ()
      n805 = global write "G_SEN.vi" "Lane_R_V"(w1116) -> ()
      n806 = global write "G_SEN.vi" "vision lane width"(3.5 ("vision lane width")) -> ()
      n807 = local write "NaN/Path/Refnum?"(FALSE ("NaN/Path/Refnum?")) -> ()
    }
  }
